vi "Process CAN Frame.vi"(10 "CAN frame":T1 {"type" items=["CAN Data", "CAN Remote"]; "identifier" format="%.0x"}) -> ()   [LabVIEW 2015]
uses:
  <vilib>/RioEmbeddedCAN/RioEmbeddedCAN.llb/CANFrameControl.ctl
  Dashboard/DashDriverInputs.ctl
  MC/MC Temp 1.ctl
  MC/MC Temp 2.ctl
  MC/MC Temp 3.ctl
  MC/MC Position.ctl
  MC/MC Current.ctl
  MC/MC Voltage.ctl
  MC/MC Flux.ctl
  MC/MC Internal Voltages.ctl
  MC/MC State.ctl
  Inverter States.ctl
  Inverter Run Modes.ctl
  VSM States.ctl
  MC/MC Faults.ctl
  MC/MC Torque.ctl
  MC/MC Mod Index and Flux Weakening.ctl
  Global Data.vi
panel:
  in  "Log Unique IDs":bool
  in  "Reset Array":bool
  out "Array":u32[](array[numeric])
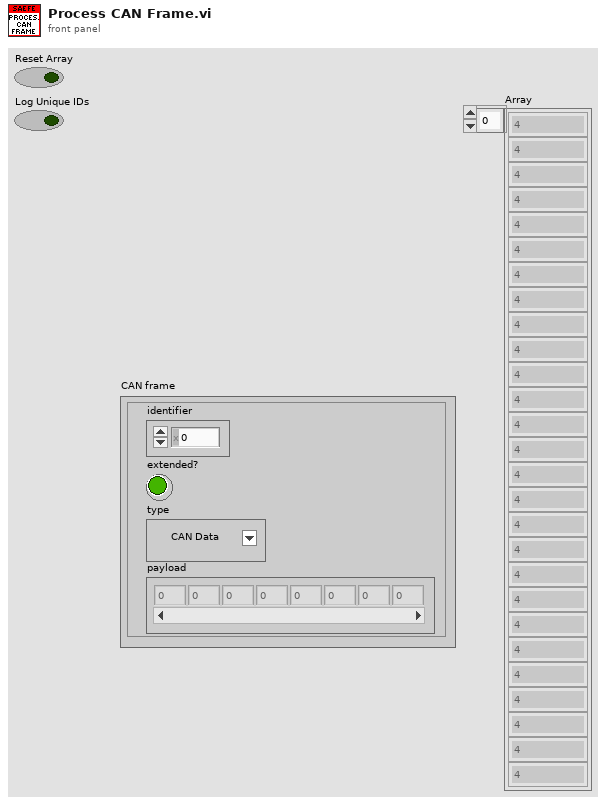
[diagram p1: front panel]
types:
  T1 = typedef "CANFrameControl.ctl" = cluster{"identifier":u32, "extended?":bool, "type":u8, "payload":u8[]}
  T2 = typedef "DashDriverInputs.ctl" = cluster{"ButtonsBitArray":u8, "NRedRotary":u8, "NYellowRotary":u8, "NBlackRotary":u8}
  T3 = typedef "MC Temp 1.ctl" = cluster{"TMCModuleA":dbl, "TMCModuleB":dbl, "TMCModuleC":dbl, "TMCGateDriver":dbl}
  T4 = typedef "MC Temp 2.ctl" = cluster{"TMCControlBoard":dbl, "TMCRTD1":dbl, "TMCRTD2":dbl, "TMCRTD3":dbl}
  T5 = typedef "MC Temp 3.ctl" = cluster{"TMCRTD4":dbl, "TMCRTD5":dbl, "TMotor":dbl, "MTorqueShudder":dbl}
  T6 = typedef "MC Position.ctl" = cluster{"aMotor":dbl, "nMotor":dbl, "fMCOutput":dbl, "aDeltaResolverFilt":dbl}
  T7 = typedef "MC Current.ctl" = cluster{"IMCPhaseA":dbl, "IMCPhaseB":dbl, "IMCPhaseC":dbl, "IMCBatteryCalc":dbl}
  T8 = typedef "MC Voltage.ctl" = cluster{"VMCPhaseAB":dbl, "VMCPhaseBC":dbl, "VMCOutput":dbl, "VMCBattery":dbl}
  T9 = typedef "MC Flux.ctl" = cluster{"IMCFluxCommand":dbl, "IMCFluxFeedback":dbl, "IMC_Id":dbl, "IMC_Iq":dbl}
  T10 = typedef "MC Internal Voltages.ctl" = cluster{"VMCRef1_5":dbl, "VMCRef2_5":dbl, "VMCRef5":dbl, "VMCRef12":dbl}
  T11 = typedef "MC State.ctl" = cluster{"eMCInverterState":T12, "eMCInverterRunMode":T13, "eMCInverterCommandMode":enum16{"CAN Mode", "VSM Mode"}, "bMCInverterEnable":bool, "bMCInverterEnableLockout":bool, "bMCDirectionForward":bool, "eMCVSMState":T14, "bMCRelay1":bool, "bMCRelay2":bool, "bMCRelay3":bool, "bMCRelay4":bool}
  T12 = typedef "Inverter States.ctl" = enum16{"Power On", "Stop", "Open Loop", "Closed Loop", "Wait", "Internal", "Idle Run", "Idle Stop", ""}
  T13 = typedef "Inverter Run Modes.ctl" = enum16{"Torque Mode", "Speed Mode"}
  T14 = typedef "VSM States.ctl" = enum16{"VSM Start", "Pre-Charge Init", "Pre-Charge Active", "Pre-Charge Complete", "VSM Wait", "VSM Ready", "Motor Running", "Blink Fault Code", "Shutdown in Process", "Recycle Power"}
  T15 = typedef "MC Faults.ctl" = cluster{"MC Fault":cluster{"Over-Speed":bool, "Over-Current":bool, "Over-Voltage":bool, "Inverter Over-Temp":bool, "Direction Command":bool, "Inverter Response Time-Out":bool, "Desat Fault":bool, "Hardware Over-Current":bool, "Under-Voltage":bool, "CAN Command Message Lost":bool, "Motor Over-Temp":bool, "Module A Over-Temp":bool, "Module B Over-Temp":bool, "Module C Over-Temp":bool, "PCB Over-Temp":bool, "Gate Driver 1 Over-Temp":bool, "Gate Driver 2 Over-Temp":bool, "Gate Drive 3 Over-Temp":bool, "Current Sensor Fault":bool, "Resolver Not Connected":bool}, "MC Post":u32, "MC RUN":u32}
  T16 = typedef "MC Torque.ctl" = cluster{"MMCRequested":dbl, "MMCFeedback":dbl, "tMCElapsed":u32}
  T17 = typedef "MC Mod Index and Flux Weakening.ctl" = cluster{"NMCModulationIndex":dbl, "IMCFluxWeakeningOutput":dbl, "IMCIdCommand":dbl, "IMCIqCommand":dbl}
  T18 = cluster{"Over-Speed":bool, "Over-Current":bool, "Over-Voltage":bool, "Inverter Over-Temp":bool, "Direction Command":bool, "Inverter Response Time-Out":bool, "Desat Fault":bool, "Hardware Over-Current":bool, "Under-Voltage":bool, "CAN Command Message Lost":bool, "Motor Over-Temp":bool, "Module A Over-Temp":bool, "Module B Over-Temp":bool, "Module C Over-Temp":bool, "PCB Over-Temp":bool, "Gate Driver 1 Over-Temp":bool, "Gate Driver 2 Over-Temp":bool, "Gate Drive 3 Over-Temp":bool, "Current Sensor Fault":bool, "Resolver Not Connected":bool}
  T19 = typedef "BMS Telemetry.ctl" = cluster{"bBMSIgnition":bool, "bBMSChargerMains":bool, "bBMSFastCharge":bool, "bBMSChargerEnabled":bool, "eBMSCarState":enum16{"Off", "On, Not Charging", "Charging", "Charging Finished", "Charging Error"}, "eBMSChargingState":enum16{"Disconnected", "Pre-charging", "Main Charging", "Balancing", "Charging Finished OK", "Charging Error"}, "tBMSChargeStage":u16, "eBMSLastChargeError":enum16{"No Error", "No Cell Communication", "No Cell Communication - Non CAN Charger", "Maximum charging stage duration expired", "Cell Communication Lost during Charge", "Cannot set balancing voltage", "Cell temps too high", "No Comms so can't determine temp", "# of Cells Mismatch", "Cells Overvoltage", "Cell Protection Event occured."}, "NBMSNumCells":u8, "bBMSUnderVProtection":bool, "bBMSOverVProtection":bool, "bBMSOverTProtection":bool, "bBMSLeakageProtection":bool, "bBMSNoCellCommsError":bool, "bBMSLowVReduction":bool, "bBMSHighTReduction":bool, "VCellMin":dbl, "VCellMax":dbl, "VCellMean":dbl, "VTotal":dbl, "TCellMin":dbl, "TCellMax":dbl, "TCellMean":dbl, "VCells":cluster{"[51]":dbl, "[53]":dbl, "[54]":dbl, "[55]":dbl, "[56]":dbl, "[57]":dbl, "[58]":dbl, "[59]":dbl, "[60]":dbl, "[61]":dbl, "[62]":dbl, "[63]":dbl, "[64]":dbl, "[65]":dbl, "[66]":dbl, "[67]":dbl, "[34]":dbl, "[35]":dbl, "[36]":dbl, "[37]":dbl, "[38]":dbl, "[39]":dbl, "[40]":dbl, "[41]":dbl, "[42]":dbl, "[43]":dbl, "[44]":dbl, "[45]":dbl, "[46]":dbl, "[47]":dbl, "[48]":dbl, "[49]":dbl, "[50]":dbl, "[17]":dbl, "[18]":dbl, "[19]":dbl, "[20]":dbl, "[21]":dbl, "[22]":dbl, "[23]":dbl, "[24]":dbl, "[25]":dbl, "[26]":dbl, "[27]":dbl, "[28]":dbl, "[29]":dbl, "[30]":dbl, "[31]":dbl, "[32]":dbl, "[33]":dbl, "[0]":dbl, "[1]":dbl, "[2]":dbl, "[3]":dbl, "[4]":dbl, "[5]":dbl, "[6]":dbl, "[7]":dbl, "[8]":dbl, "[9]":dbl, "[10]":dbl, "[11]":dbl, "[12]":dbl, "[13]":dbl, "[14]":dbl, "[15]":dbl, "[16]":dbl, "[52] 2":dbl}, "TBMSCells":cluster{"[55]":dbl, "[56]":dbl, "[57]":dbl, "[58]":dbl, "[59]":dbl, "[60]":dbl, "[61]":dbl, "[62]":dbl, "[63]":dbl, "[64]":dbl, "[65]":dbl, "[66]":dbl, "[67]":dbl, "[68]":dbl, "[69]":dbl, "[70]":dbl, "[17]":dbl, "[38]":dbl, "[39]":dbl, "[40]":dbl, "[41]":dbl, "[42]":dbl, "[43]":dbl, "[44]":dbl, "[45]":dbl, "[46]":dbl, "[47]":dbl, "[48]":dbl, "[49]":dbl, "[50]":dbl, "[51]":dbl, "[52]":dbl, "[53]":dbl, "[54]":dbl, "[21]":dbl, "[22]":dbl, "[23]":dbl, "[24]":dbl, "[25]":dbl, "[26]":dbl, "[27]":dbl, "[28]":dbl, "[29]":dbl, "[30]":dbl, "[31]":dbl, "[32]":dbl, "[33]":dbl, "[34]":dbl, "[35]":dbl, "[36]":dbl, "[37]":dbl, "[0]":dbl, "[1]":dbl, "[2]":dbl, "[3]":dbl, "[4]":dbl, "[5]":dbl, "[6]":dbl, "[7]":dbl, "[8]":dbl, "[9]":dbl, "[10]":dbl, "[11]":dbl, "[12]":dbl, "[13]":dbl, "[14]":dbl, "[15]":dbl, "[16]":dbl}, "bChargerConnected":bool, "VChargerSetpoint":dbl, "IChargerSetpoint":dbl, "VChargerActual":dbl, "IChargerActual":dbl, "BCells":cluster{"[51]":dbl, "[52]":dbl, "[53]":dbl, "[54]":dbl, "[55]":dbl, "[56]":dbl, "[57]":dbl, "[58]":dbl, "[59]":dbl, "[60]":dbl, "[61]":dbl, "[62]":dbl, "[63]":dbl, "[64]":dbl, "[65]":dbl, "[66]":dbl, "[67]":dbl, "[34]":dbl, "[35]":dbl, "[36]":dbl, "[37]":dbl, "[38]":dbl, "[39]":dbl, "[40]":dbl, "[41]":dbl, "[42]":dbl, "[43]":dbl, "[44]":dbl, "[45]":dbl, "[46]":dbl, "[47]":dbl, "[48]":dbl, "[49]":dbl, "[50]":dbl, "[17]":dbl, "[18]":dbl, "[19]":dbl, "[20]":dbl, "[21]":dbl, "[22]":dbl, "[23]":dbl, "[24]":dbl, "[25]":dbl, "[26]":dbl, "[27]":dbl, "[28]":dbl, "[29]":dbl, "[30]":dbl, "[31]":dbl, "[32]":dbl, "[33]":dbl, "[0]":dbl, "[1]":dbl, "[2]":dbl, "[3]":dbl, "[4]":dbl, "[5]":dbl, "[6]":dbl, "[7]":dbl, "[8]":dbl, "[9]":dbl, "[10]":dbl, "[11]":dbl, "[12]":dbl, "[13]":dbl, "[14]":dbl, "[15]":dbl, "[16]":dbl}, "bNewVCellMinSample":bool, "Battery Temp":cluster{"[0]":dbl, "[1]":dbl, "[2]":dbl, "[3]":dbl, "[4]":dbl, "[5]":dbl, "[6]":dbl, "[7]":dbl, "[8]":dbl, "[9]":dbl, "[10]":dbl, "[11]":dbl, "[12]":dbl, "[13]":dbl, "[14]":dbl, "[15]":dbl, "[16]":dbl, "[17]":dbl, "[18]":dbl, "[19]":dbl, "[20]":dbl, "[21]":dbl, "[22]":dbl, "[23]":dbl, "[24]":dbl, "[25]":dbl, "[26]":dbl, "[27]":dbl, "[28]":dbl, "[29]":dbl, "[30]":dbl, "[31]":dbl, "[32]":dbl, "[33]":dbl, "[34]":dbl, "[35]":dbl, "[36]":dbl, "[37]":dbl, "[38]":dbl, "[39]":dbl, "[40]":dbl, "[41]":dbl, "[42]":dbl, "[43]":dbl, "[44]":dbl, "[45]":dbl, "[46]":dbl, "[47]":dbl, "[48]":dbl, "[49]":dbl, "[50]":dbl, "[51]":dbl, "[52]":dbl, "[53]":dbl, "[54]":dbl, "[55]":dbl, "[56]":dbl, "[57]":dbl, "[58]":dbl, "[59]":dbl, "[60]":dbl, "[61]":dbl, "[62]":dbl, "[63]":dbl, "[64]":dbl, "[65]":dbl, "[66]":dbl, "[67]":dbl, "[68]":dbl, "[69]":dbl, "[71]":dbl, "[70]":dbl, "[0] 2":dbl, "[1] 2":dbl, "[2] 2":dbl, "[3] 2":dbl, "[4] 2":dbl, "[5] 2":dbl, "[6] 2":dbl, "[7] 2":dbl, "[8] 2":dbl, "[9] 2":dbl, "[10] 2":dbl, "[11] 2":dbl, "[12] 2":dbl, "[13] 2":dbl, "[14] 2":dbl, "[15] 2":dbl, "[16] 2":dbl, "[17] 2":dbl, "[18] 2":dbl, "[19] 2":dbl, "[20] 2":dbl, "[21] 2":dbl, "[22] 2":dbl, "[23] 2":dbl, "[24] 2":dbl, "[25] 2":dbl, "[26] 2":dbl, "[27] 2":dbl, "[28] 2":dbl, "[29] 2":dbl, "[30] 2":dbl, "[31] 2":dbl, "[32] 2":dbl, "[33] 2":dbl, "[34] 2":dbl, "[35] 2":dbl, "[36] 2":dbl, "[37] 2":dbl, "[38] 2":dbl, "[39] 2":dbl, "[40] 2":dbl, "[41] 2":dbl, "[42] 2":dbl, "[43] 2":dbl, "[44] 2":dbl, "[45] 2":dbl, "[46] 2":dbl, "[47] 2":dbl, "[48] 2":dbl, "[49] 2":dbl, "[50] 2":dbl, "[51] 2":dbl, "[52] 3":dbl, "[53] 2":dbl, "[54] 2":dbl, "[55] 2":dbl, "[56] 2":dbl, "[57] 2":dbl, "[58] 2":dbl, "[59] 2":dbl, "[60] 2":dbl, "[61] 2":dbl, "[62] 2":dbl, "[63] 2":dbl, "[64] 2":dbl, "[65] 2":dbl, "[66] 2":dbl, "[67] 2":dbl, "[68]2":dbl, "[69]2":dbl, "[70]2":dbl, "[71]2":dbl, "[0] 3":dbl, "[1] 3":dbl, "[2] 3":dbl, "[3] 3":dbl, "[4] 3":dbl, "[5] 3":dbl, "[6] 3":dbl, "[7] 3":dbl, "[8] 3":dbl, "[9] 3":dbl, "[10] 3":dbl, "[11] 3":dbl, "[12] 3":dbl, "[13] 3":dbl, "[14] 3":dbl, "[15] 3":dbl, "[16] 3":dbl, "[17] 3":dbl, "[18] 3":dbl, "[19] 3":dbl, "[20] 3":dbl, "[21] 3":dbl, "[22] 3":dbl, "[23] 3":dbl, "[24] 3":dbl, "[25] 3":dbl, "[26] 3":dbl, "[27] 3":dbl, "[28] 3":dbl, "[29] 3":dbl, "[30] 3":dbl, "[31] 3":dbl, "[32] 3":dbl, "[33] 3":dbl, "[34] 3":dbl, "[35] 3":dbl, "[36] 3":dbl, "[37] 3":dbl, "[38] 3":dbl, "[39] 3":dbl, "[40] 3":dbl, "[41] 3":dbl, "[42] 3":dbl, "[43] 3":dbl, "[44] 3":dbl, "[45] 3":dbl, "[46] 3":dbl, "[47] 3":dbl, "[48] 3":dbl, "[49] 3":dbl, "[50] 3":dbl, "[51] 3":dbl, "[52] 4":dbl, "[53] 3":dbl, "[54] 3":dbl, "[55] 3":dbl, "[56] 3":dbl, "[57] 3":dbl, "[58] 3":dbl, "[59] 3":dbl, "[60] 3":dbl, "[61] 3":dbl, "[62] 3":dbl, "[63] 3":dbl, "[64] 3":dbl, "[65] 3":dbl, "[66] 3":dbl, "[67] 3":dbl, "[68]3":dbl, "[69]3":dbl, "[70]3":dbl, "[71]3":dbl, "[4] 4":dbl, "[5] 4":dbl, "[6] 4":dbl, "[7] 4":dbl, "[8] 4":dbl, "[9] 4":dbl, "[10] 4":dbl, "[11] 4":dbl, "[12] 4":dbl, "[13] 4":dbl, "[14] 4":dbl, "[15] 4":dbl, "[16] 4":dbl, "[17] 4":dbl, "[18] 4":dbl, "[19] 4":dbl, "[20] 4":dbl, "[21] 4":dbl, "[22] 4":dbl, "[23] 4":dbl, "[24] 4":dbl, "[25] 4":dbl, "[26] 4":dbl, "[27] 4":dbl, "[28] 4":dbl, "[29] 4":dbl, "[30] 4":dbl, "[31] 4":dbl, "[32] 4":dbl, "[33] 4":dbl, "[17] 9":dbl, "[0] 9":dbl, "[51] 8":dbl, "[34] 8":dbl, "[17] 8":dbl, "[0] 8":dbl, "[34] 4":dbl, "[35] 4":dbl, "[36] 4":dbl, "[37] 4":dbl, "[38] 4":dbl, "[39] 4":dbl, "[40] 4":dbl, "[41] 4":dbl, "[42] 4":dbl, "[43] 4":dbl, "[44] 4":dbl, "[45] 4":dbl, "[46] 4":dbl, "[47] 4":dbl, "[48] 4":dbl, "[49] 4":dbl, "[50] 4":dbl, "[34] 9":dbl, "[51] 4":dbl, "[52] 5":dbl, "[53] 4":dbl, "[54] 4":dbl, "[55] 4":dbl, "[56] 4":dbl, "[57] 4":dbl, "[58] 4":dbl, "[59] 4":dbl, "[60] 4":dbl, "[61] 4":dbl, "[62] 4":dbl, "[63] 4":dbl, "[64] 4":dbl, "[65] 4":dbl, "[66] 4":dbl, "[67] 4":dbl, "[51] 9":dbl}, "TBMSMax":dbl, "TBMSMin":dbl, "TBMSMean":dbl}
  T20 = enum16{"Off", "On, Not Charging", "Charging", "Charging Finished", "Charging Error"}
  T21 = enum16{"Disconnected", "Pre-charging", "Main Charging", "Balancing", "Charging Finished OK", "Charging Error"}
  T22 = cluster{"[51]":dbl, "[53]":dbl, "[54]":dbl, "[55]":dbl, "[56]":dbl, "[57]":dbl, "[58]":dbl, "[59]":dbl, "[60]":dbl, "[61]":dbl, "[62]":dbl, "[63]":dbl, "[64]":dbl, "[65]":dbl, "[66]":dbl, "[67]":dbl, "[34]":dbl, "[35]":dbl, "[36]":dbl, "[37]":dbl, "[38]":dbl, "[39]":dbl, "[40]":dbl, "[41]":dbl, "[42]":dbl, "[43]":dbl, "[44]":dbl, "[45]":dbl, "[46]":dbl, "[47]":dbl, "[48]":dbl, "[49]":dbl, "[50]":dbl, "[17]":dbl, "[18]":dbl, "[19]":dbl, "[20]":dbl, "[21]":dbl, "[22]":dbl, "[23]":dbl, "[24]":dbl, "[25]":dbl, "[26]":dbl, "[27]":dbl, "[28]":dbl, "[29]":dbl, "[30]":dbl, "[31]":dbl, "[32]":dbl, "[33]":dbl, "[0]":dbl, "[1]":dbl, "[2]":dbl, "[3]":dbl, "[4]":dbl, "[5]":dbl, "[6]":dbl, "[7]":dbl, "[8]":dbl, "[9]":dbl, "[10]":dbl, "[11]":dbl, "[12]":dbl, "[13]":dbl, "[14]":dbl, "[15]":dbl, "[16]":dbl, "[52] 2":dbl}
  T23 = cluster{"VCells[0]":dbl, "VCells[1]":dbl, "VCells[2]":dbl, "VCells[3]":dbl, "VCells[4]":dbl, "VCells[5]":dbl, "VCells[6]":dbl, "VCells[7]":dbl, "VCells[8]":dbl, "VCells[9]":dbl, "VCells[10]":dbl, "VCells[11]":dbl, "VCells[12]":dbl, "VCells[13]":dbl, "VCells[14]":dbl, "VCells[15]":dbl, "VCells[16]":dbl, "VCells[17]":dbl, "VCells[18]":dbl, "VCells[19]":dbl, "VCells[20]":dbl, "VCells[21]":dbl, "VCells[22]":dbl, "VCells[23]":dbl, "VCells[24]":dbl, "VCells[25]":dbl, "VCells[26]":dbl, "VCells[27]":dbl, "VCells[28]":dbl, "VCells[29]":dbl, "VCells[30]":dbl, "VCells[31]":dbl, "VCells[32]":dbl, "VCells[33]":dbl, "VCells[34]":dbl, "VCells[35]":dbl, "VCells[36]":dbl, "VCells[37]":dbl, "VCells[38]":dbl, "VCells[39]":dbl, "VCells[40]":dbl, "VCells[41]":dbl, "VCells[42]":dbl, "VCells[43]":dbl, "VCells[44]":dbl, "VCells[45]":dbl, "VCells[46]":dbl, "VCells[47]":dbl, "VCells[48]":dbl, "VCells[49]":dbl, "VCells[50]":dbl, "VCells[51]":dbl, "VCells[52]":dbl, "VCells[53]":dbl, "VCells[54]":dbl, "VCells[55]":dbl, "VCells[56]":dbl, "VCells[57]":dbl, "VCells[58]":dbl, "VCells[59]":dbl, "VCells[60]":dbl, "VCells[61]":dbl, "VCells[62]":dbl, "VCells[63]":dbl, "VCells[64]":dbl, "VCells[65]":dbl, "VCells[66]":dbl, "VCells[67]":dbl}
  T24 = cluster{"[55]":dbl, "[56]":dbl, "[57]":dbl, "[58]":dbl, "[59]":dbl, "[60]":dbl, "[61]":dbl, "[62]":dbl, "[63]":dbl, "[64]":dbl, "[65]":dbl, "[66]":dbl, "[67]":dbl, "[68]":dbl, "[69]":dbl, "[70]":dbl, "[17]":dbl, "[38]":dbl, "[39]":dbl, "[40]":dbl, "[41]":dbl, "[42]":dbl, "[43]":dbl, "[44]":dbl, "[45]":dbl, "[46]":dbl, "[47]":dbl, "[48]":dbl, "[49]":dbl, "[50]":dbl, "[51]":dbl, "[52]":dbl, "[53]":dbl, "[54]":dbl, "[21]":dbl, "[22]":dbl, "[23]":dbl, "[24]":dbl, "[25]":dbl, "[26]":dbl, "[27]":dbl, "[28]":dbl, "[29]":dbl, "[30]":dbl, "[31]":dbl, "[32]":dbl, "[33]":dbl, "[34]":dbl, "[35]":dbl, "[36]":dbl, "[37]":dbl, "[0]":dbl, "[1]":dbl, "[2]":dbl, "[3]":dbl, "[4]":dbl, "[5]":dbl, "[6]":dbl, "[7]":dbl, "[8]":dbl, "[9]":dbl, "[10]":dbl, "[11]":dbl, "[12]":dbl, "[13]":dbl, "[14]":dbl, "[15]":dbl, "[16]":dbl}
  T25 = cluster{"TBMSCells[0]":dbl, "TBMSCells[1]":dbl, "TBMSCells[2]":dbl, "TBMSCells[3]":dbl, "TBMSCells[4]":dbl, "TBMSCells[5]":dbl, "TBMSCells[6]":dbl, "TBMSCells[7]":dbl, "TBMSCells[8]":dbl, "TBMSCells[9]":dbl, "TBMSCells[10]":dbl, "TBMSCells[11]":dbl, "TBMSCells[12]":dbl, "TBMSCells[13]":dbl, "TBMSCells[14]":dbl, "TBMSCells[15]":dbl, "TBMSCells[16]":dbl, "TBMSCells[17]":dbl, "TBMSCells[18]":dbl, "TBMSCells[19]":dbl, "TBMSCells[20]":dbl, "TBMSCells[21]":dbl, "TBMSCells[22]":dbl, "TBMSCells[23]":dbl, "TBMSCells[24]":dbl, "TBMSCells[25]":dbl, "TBMSCells[26]":dbl, "TBMSCells[27]":dbl, "TBMSCells[28]":dbl, "TBMSCells[29]":dbl, "TBMSCells[30]":dbl, "TBMSCells[31]":dbl, "TBMSCells[32]":dbl, "TBMSCells[33]":dbl, "TBMSCells[34]":dbl, "TBMSCells[35]":dbl, "TBMSCells[36]":dbl, "TBMSCells[37]":dbl, "TBMSCells[38]":dbl, "TBMSCells[39]":dbl, "TBMSCells[40]":dbl, "TBMSCells[41]":dbl, "TBMSCells[42]":dbl, "TBMSCells[43]":dbl, "TBMSCells[44]":dbl, "TBMSCells[45]":dbl, "TBMSCells[46]":dbl, "TBMSCells[47]":dbl, "TBMSCells[48]":dbl, "TBMSCells[49]":dbl, "TBMSCells[50]":dbl, "TBMSCells[51]":dbl, "TBMSCells[52]":dbl, "TBMSCells[53]":dbl, "TBMSCells[54]":dbl, "TBMSCells[55]":dbl, "TBMSCells[56]":dbl, "TBMSCells[57]":dbl, "TBMSCells[58]":dbl, "TBMSCells[59]":dbl, "TBMSCells[60]":dbl, "TBMSCells[61]":dbl, "TBMSCells[62]":dbl, "TBMSCells[63]":dbl, "TBMSCells[64]":dbl, "TBMSCells[65]":dbl, "TBMSCells[66]":dbl, "TBMSCells[67]":dbl}
  T26 = cluster{"[51]":dbl, "[52]":dbl, "[53]":dbl, "[54]":dbl, "[55]":dbl, "[56]":dbl, "[57]":dbl, "[58]":dbl, "[59]":dbl, "[60]":dbl, "[61]":dbl, "[62]":dbl, "[63]":dbl, "[64]":dbl, "[65]":dbl, "[66]":dbl, "[67]":dbl, "[34]":dbl, "[35]":dbl, "[36]":dbl, "[37]":dbl, "[38]":dbl, "[39]":dbl, "[40]":dbl, "[41]":dbl, "[42]":dbl, "[43]":dbl, "[44]":dbl, "[45]":dbl, "[46]":dbl, "[47]":dbl, "[48]":dbl, "[49]":dbl, "[50]":dbl, "[17]":dbl, "[18]":dbl, "[19]":dbl, "[20]":dbl, "[21]":dbl, "[22]":dbl, "[23]":dbl, "[24]":dbl, "[25]":dbl, "[26]":dbl, "[27]":dbl, "[28]":dbl, "[29]":dbl, "[30]":dbl, "[31]":dbl, "[32]":dbl, "[33]":dbl, "[0]":dbl, "[1]":dbl, "[2]":dbl, "[3]":dbl, "[4]":dbl, "[5]":dbl, "[6]":dbl, "[7]":dbl, "[8]":dbl, "[9]":dbl, "[10]":dbl, "[11]":dbl, "[12]":dbl, "[13]":dbl, "[14]":dbl, "[15]":dbl, "[16]":dbl}
  T27 = cluster{"BCells[0]":dbl, "BCells[1]":dbl, "BCells[2]":dbl, "BCells[3]":dbl, "BCells[4]":dbl, "BCells[5]":dbl, "BCells[6]":dbl, "BCells[7]":dbl, "BCells[8]":dbl, "BCells[9]":dbl, "BCells[10]":dbl, "BCells[11]":dbl, "BCells[12]":dbl, "BCells[13]":dbl, "BCells[14]":dbl, "BCells[15]":dbl, "BCells[16]":dbl, "BCells[17]":dbl, "BCells[18]":dbl, "BCells[19]":dbl, "BCells[20]":dbl, "BCells[21]":dbl, "BCells[22]":dbl, "BCells[23]":dbl, "BCells[24]":dbl, "BCells[25]":dbl, "BCells[26]":dbl, "BCells[27]":dbl, "BCells[28]":dbl, "BCells[29]":dbl, "BCells[30]":dbl, "BCells[31]":dbl, "BCells[32]":dbl, "BCells[33]":dbl, "BCells[34]":dbl, "BCells[35]":dbl, "BCells[36]":dbl, "BCells[37]":dbl, "BCells[38]":dbl, "BCells[39]":dbl, "BCells[40]":dbl, "BCells[41]":dbl, "BCells[42]":dbl, "BCells[43]":dbl, "BCells[44]":dbl, "BCells[45]":dbl, "BCells[46]":dbl, "BCells[47]":dbl, "BCells[48]":dbl, "BCells[49]":dbl, "BCells[50]":dbl, "BCells[51]":dbl, "BCells[52]":dbl, "BCells[53]":dbl, "BCells[54]":dbl, "BCells[55]":dbl, "BCells[56]":dbl, "BCells[57]":dbl, "BCells[58]":dbl, "BCells[59]":dbl, "BCells[60]":dbl, "BCells[61]":dbl, "BCells[62]":dbl, "BCells[63]":dbl, "BCells[64]":dbl, "BCells[65]":dbl, "BCells[66]":dbl, "BCells[67]":dbl}
  T28 = cluster{dbl, dbl, dbl, dbl, dbl, dbl, dbl, dbl, dbl, dbl, dbl, dbl, dbl, dbl, dbl, dbl, dbl, dbl, dbl, dbl, dbl, dbl, dbl, dbl, dbl, dbl, dbl, dbl, dbl, dbl, dbl, dbl, dbl, dbl, dbl, dbl, dbl, dbl, dbl, dbl, dbl, dbl, dbl, dbl, dbl, dbl, dbl, dbl, dbl, dbl, dbl, dbl, dbl, dbl, dbl, dbl, dbl, dbl, dbl, dbl, dbl, dbl, dbl, dbl, dbl, dbl, dbl, dbl, dbl, dbl, dbl, dbl, dbl, dbl, dbl, dbl, dbl, dbl, dbl, dbl, dbl, dbl, dbl, dbl, dbl, dbl, dbl, dbl, dbl, dbl, dbl, dbl, dbl, dbl, dbl, dbl, dbl, dbl, dbl, dbl, dbl, dbl, dbl, dbl, dbl, dbl, dbl, dbl, dbl, dbl, dbl, dbl, dbl, dbl, dbl, dbl, dbl, dbl, dbl, dbl, dbl, dbl, dbl, dbl, dbl, dbl, dbl, dbl, dbl, dbl, dbl, dbl, dbl, dbl, dbl, dbl, dbl, dbl, dbl, dbl, dbl, dbl, dbl, dbl, dbl, dbl, dbl, dbl, dbl, dbl, dbl, dbl, dbl, dbl, dbl, dbl, dbl, dbl, dbl, dbl, dbl, dbl, dbl, dbl, dbl, dbl, dbl, dbl, dbl, dbl, dbl, dbl, dbl, dbl, dbl, dbl, dbl, dbl, dbl, dbl, dbl, dbl, dbl, dbl, dbl, dbl, dbl, dbl, dbl, dbl, dbl, dbl, dbl, dbl, dbl, dbl, dbl, dbl, dbl, dbl, dbl, dbl, dbl, dbl, dbl, dbl, dbl, dbl, dbl, dbl, dbl, dbl, dbl, dbl, dbl, dbl, dbl, dbl, dbl, dbl, dbl, dbl, dbl, dbl, dbl, dbl, dbl, dbl, dbl, dbl, dbl, dbl, dbl, dbl, dbl, dbl, dbl, dbl, dbl, dbl, dbl, dbl, dbl, dbl, dbl, dbl, dbl, dbl, dbl, dbl, dbl, dbl, dbl, dbl, dbl, dbl, dbl, dbl, dbl, dbl, dbl, dbl, dbl, dbl, dbl, dbl, dbl, dbl, dbl, dbl, dbl, dbl, dbl, dbl, dbl, dbl, dbl, dbl, dbl, dbl, dbl, dbl, dbl, dbl, dbl, dbl, dbl, dbl}
  T29 = cluster{"[0]":dbl, "[1]":dbl, "[2]":dbl, "[3]":dbl, "[4]":dbl, "[5]":dbl, "[6]":dbl, "[7]":dbl, "[8]":dbl, "[9]":dbl, "[10]":dbl, "[11]":dbl, "[12]":dbl, "[13]":dbl, "[14]":dbl, "[15]":dbl, "[16]":dbl, "[17]":dbl, "[18]":dbl, "[19]":dbl, "[20]":dbl, "[21]":dbl, "[22]":dbl, "[23]":dbl, "[24]":dbl, "[25]":dbl, "[26]":dbl, "[27]":dbl, "[28]":dbl, "[29]":dbl, "[30]":dbl, "[31]":dbl, "[32]":dbl, "[33]":dbl, "[34]":dbl, "[35]":dbl, "[36]":dbl, "[37]":dbl, "[38]":dbl, "[39]":dbl, "[40]":dbl, "[41]":dbl, "[42]":dbl, "[43]":dbl, "[44]":dbl, "[45]":dbl, "[46]":dbl, "[47]":dbl, "[48]":dbl, "[49]":dbl, "[50]":dbl, "[51]":dbl, "[52]":dbl, "[53]":dbl, "[54]":dbl, "[55]":dbl, "[56]":dbl, "[57]":dbl, "[58]":dbl, "[59]":dbl, "[60]":dbl, "[61]":dbl, "[62]":dbl, "[63]":dbl, "[64]":dbl, "[65]":dbl, "[66]":dbl, "[67]":dbl, "[68]":dbl, "[69]":dbl, "[71]":dbl, "[70]":dbl, "[0] 2":dbl, "[1] 2":dbl, "[2] 2":dbl, "[3] 2":dbl, "[4] 2":dbl, "[5] 2":dbl, "[6] 2":dbl, "[7] 2":dbl, "[8] 2":dbl, "[9] 2":dbl, "[10] 2":dbl, "[11] 2":dbl, "[12] 2":dbl, "[13] 2":dbl, "[14] 2":dbl, "[15] 2":dbl, "[16] 2":dbl, "[17] 2":dbl, "[18] 2":dbl, "[19] 2":dbl, "[20] 2":dbl, "[21] 2":dbl, "[22] 2":dbl, "[23] 2":dbl, "[24] 2":dbl, "[25] 2":dbl, "[26] 2":dbl, "[27] 2":dbl, "[28] 2":dbl, "[29] 2":dbl, "[30] 2":dbl, "[31] 2":dbl, "[32] 2":dbl, "[33] 2":dbl, "[34] 2":dbl, "[35] 2":dbl, "[36] 2":dbl, "[37] 2":dbl, "[38] 2":dbl, "[39] 2":dbl, "[40] 2":dbl, "[41] 2":dbl, "[42] 2":dbl, "[43] 2":dbl, "[44] 2":dbl, "[45] 2":dbl, "[46] 2":dbl, "[47] 2":dbl, "[48] 2":dbl, "[49] 2":dbl, "[50] 2":dbl, "[51] 2":dbl, "[52] 3":dbl, "[53] 2":dbl, "[54] 2":dbl, "[55] 2":dbl, "[56] 2":dbl, "[57] 2":dbl, "[58] 2":dbl, "[59] 2":dbl, "[60] 2":dbl, "[61] 2":dbl, "[62] 2":dbl, "[63] 2":dbl, "[64] 2":dbl, "[65] 2":dbl, "[66] 2":dbl, "[67] 2":dbl, "[68]2":dbl, "[69]2":dbl, "[70]2":dbl, "[71]2":dbl, "[0] 3":dbl, "[1] 3":dbl, "[2] 3":dbl, "[3] 3":dbl, "[4] 3":dbl, "[5] 3":dbl, "[6] 3":dbl, "[7] 3":dbl, "[8] 3":dbl, "[9] 3":dbl, "[10] 3":dbl, "[11] 3":dbl, "[12] 3":dbl, "[13] 3":dbl, "[14] 3":dbl, "[15] 3":dbl, "[16] 3":dbl, "[17] 3":dbl, "[18] 3":dbl, "[19] 3":dbl, "[20] 3":dbl, "[21] 3":dbl, "[22] 3":dbl, "[23] 3":dbl, "[24] 3":dbl, "[25] 3":dbl, "[26] 3":dbl, "[27] 3":dbl, "[28] 3":dbl, "[29] 3":dbl, "[30] 3":dbl, "[31] 3":dbl, "[32] 3":dbl, "[33] 3":dbl, "[34] 3":dbl, "[35] 3":dbl, "[36] 3":dbl, "[37] 3":dbl, "[38] 3":dbl, "[39] 3":dbl, "[40] 3":dbl, "[41] 3":dbl, "[42] 3":dbl, "[43] 3":dbl, "[44] 3":dbl, "[45] 3":dbl, "[46] 3":dbl, "[47] 3":dbl, "[48] 3":dbl, "[49] 3":dbl, "[50] 3":dbl, "[51] 3":dbl, "[52] 4":dbl, "[53] 3":dbl, "[54] 3":dbl, "[55] 3":dbl, "[56] 3":dbl, "[57] 3":dbl, "[58] 3":dbl, "[59] 3":dbl, "[60] 3":dbl, "[61] 3":dbl, "[62] 3":dbl, "[63] 3":dbl, "[64] 3":dbl, "[65] 3":dbl, "[66] 3":dbl, "[67] 3":dbl, "[68]3":dbl, "[69]3":dbl, "[70]3":dbl, "[71]3":dbl, "[4] 4":dbl, "[5] 4":dbl, "[6] 4":dbl, "[7] 4":dbl, "[8] 4":dbl, "[9] 4":dbl, "[10] 4":dbl, "[11] 4":dbl, "[12] 4":dbl, "[13] 4":dbl, "[14] 4":dbl, "[15] 4":dbl, "[16] 4":dbl, "[17] 4":dbl, "[18] 4":dbl, "[19] 4":dbl, "[20] 4":dbl, "[21] 4":dbl, "[22] 4":dbl, "[23] 4":dbl, "[24] 4":dbl, "[25] 4":dbl, "[26] 4":dbl, "[27] 4":dbl, "[28] 4":dbl, "[29] 4":dbl, "[30] 4":dbl, "[31] 4":dbl, "[32] 4":dbl, "[33] 4":dbl, "[17] 9":dbl, "[0] 9":dbl, "[51] 8":dbl, "[34] 8":dbl, "[17] 8":dbl, "[0] 8":dbl, "[34] 4":dbl, "[35] 4":dbl, "[36] 4":dbl, "[37] 4":dbl, "[38] 4":dbl, "[39] 4":dbl, "[40] 4":dbl, "[41] 4":dbl, "[42] 4":dbl, "[43] 4":dbl, "[44] 4":dbl, "[45] 4":dbl, "[46] 4":dbl, "[47] 4":dbl, "[48] 4":dbl, "[49] 4":dbl, "[50] 4":dbl, "[34] 9":dbl, "[51] 4":dbl, "[52] 5":dbl, "[53] 4":dbl, "[54] 4":dbl, "[55] 4":dbl, "[56] 4":dbl, "[57] 4":dbl, "[58] 4":dbl, "[59] 4":dbl, "[60] 4":dbl, "[61] 4":dbl, "[62] 4":dbl, "[63] 4":dbl, "[64] 4":dbl, "[65] 4":dbl, "[66] 4":dbl, "[67] 4":dbl, "[51] 9":dbl}
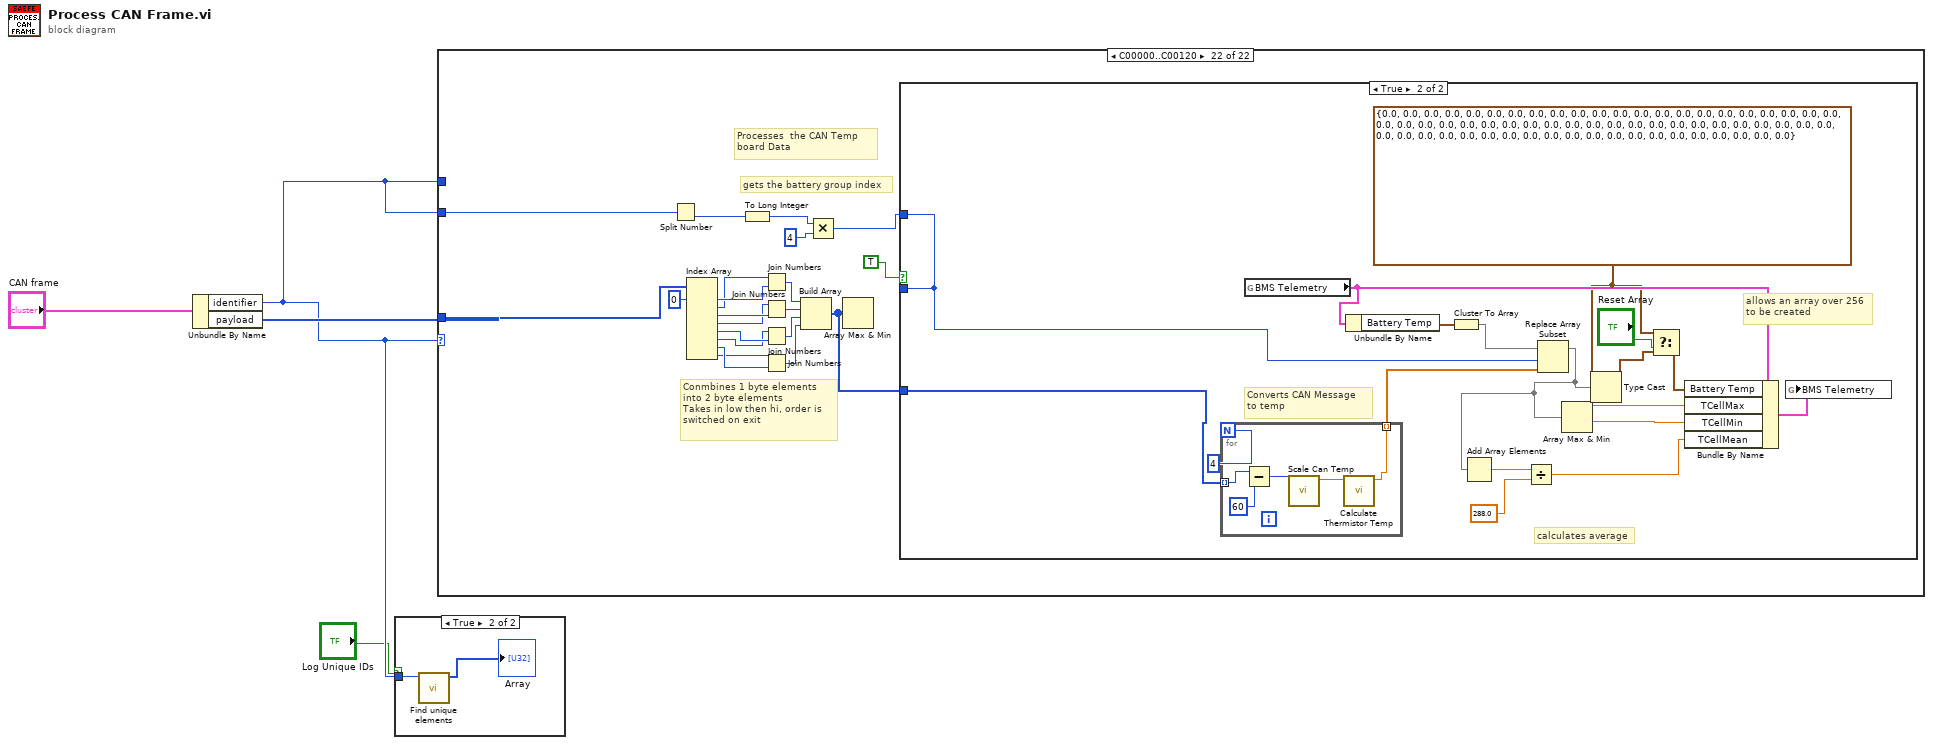
[diagram p0: block diagram]
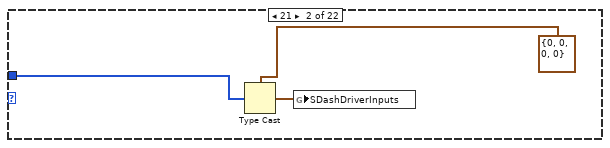
[diagram p4: hidden frame]
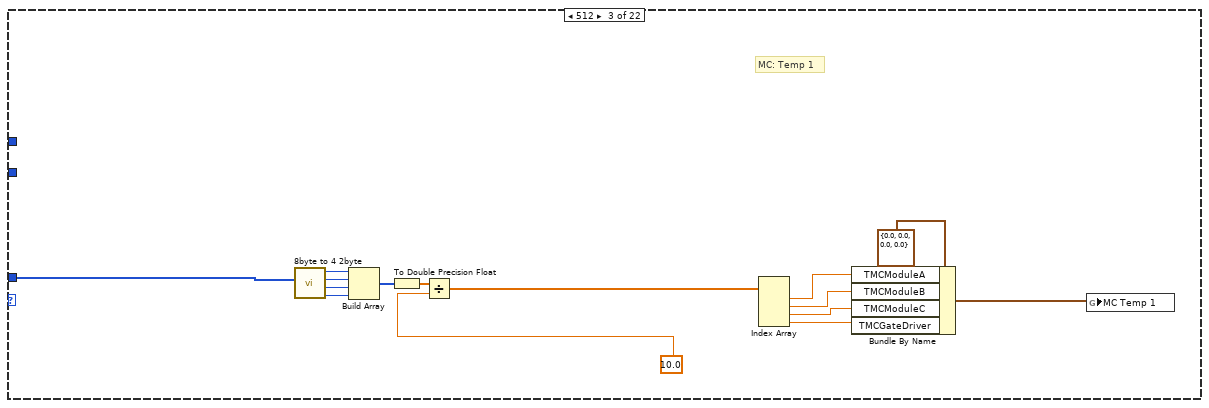
[diagram p5: hidden frame]
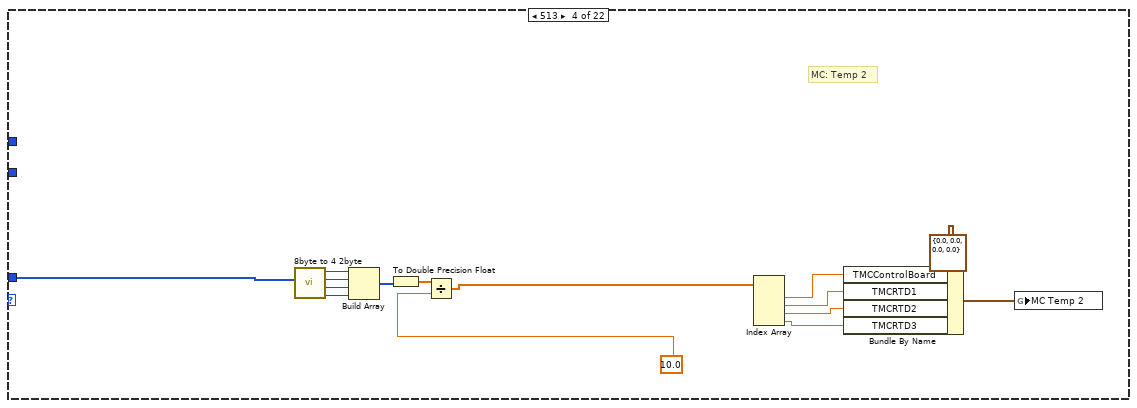
[diagram p6: hidden frame]
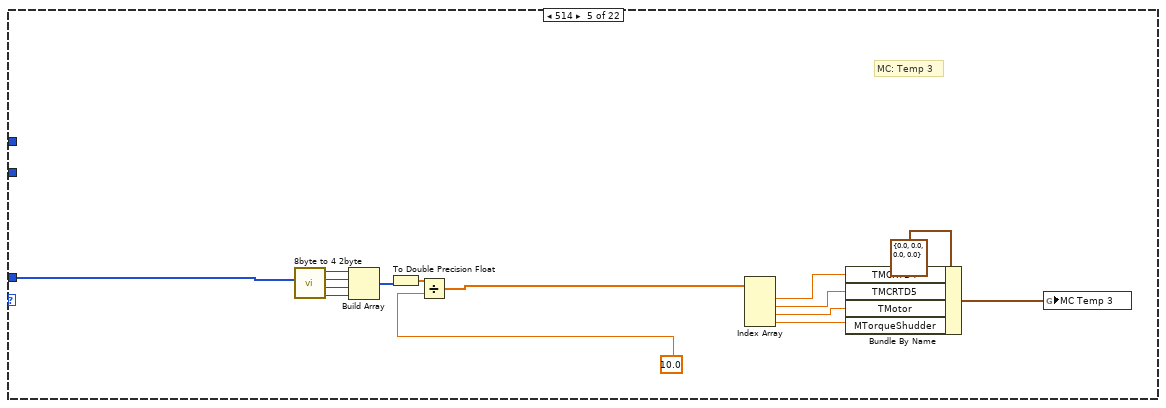
[diagram p7: hidden frame]
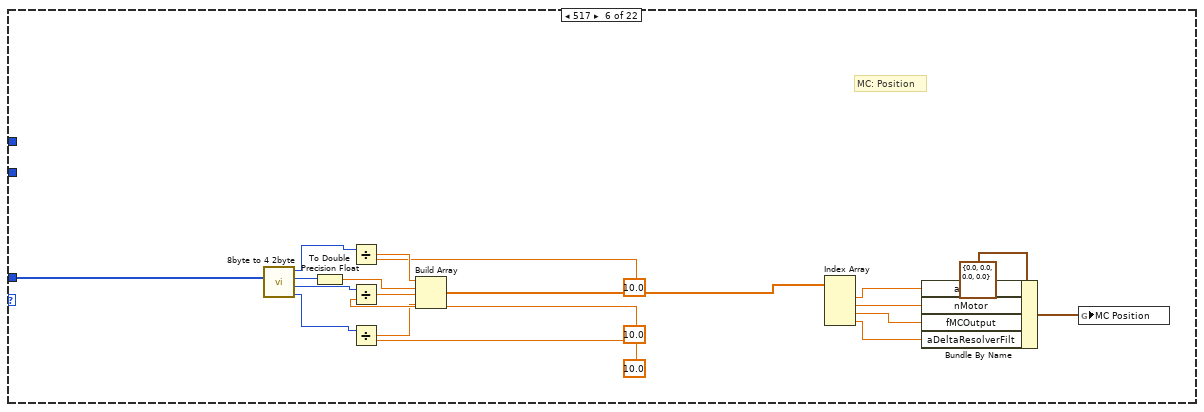
[diagram p8: hidden frame]
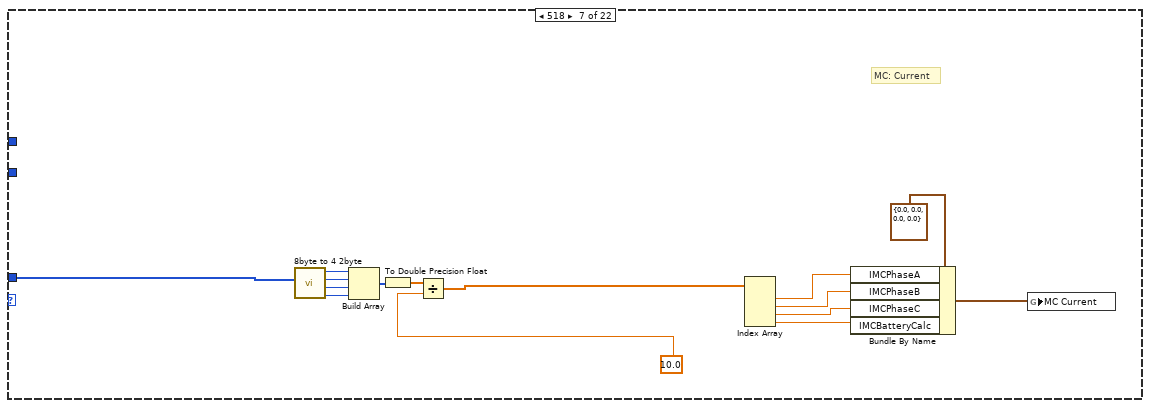
[diagram p9: hidden frame]
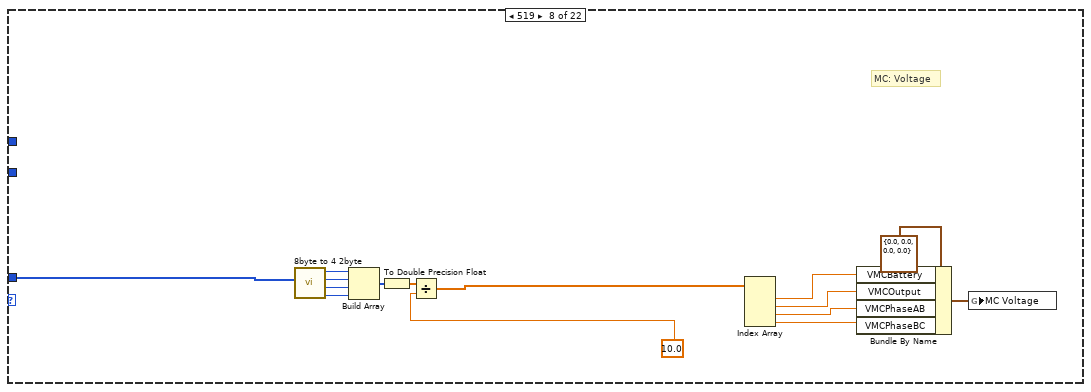
[diagram p10: hidden frame]
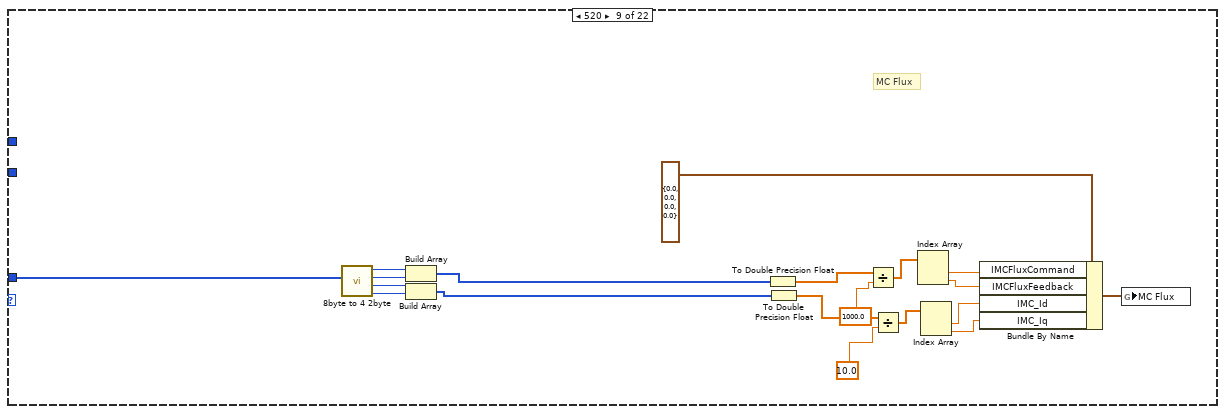
[diagram p11: hidden frame]
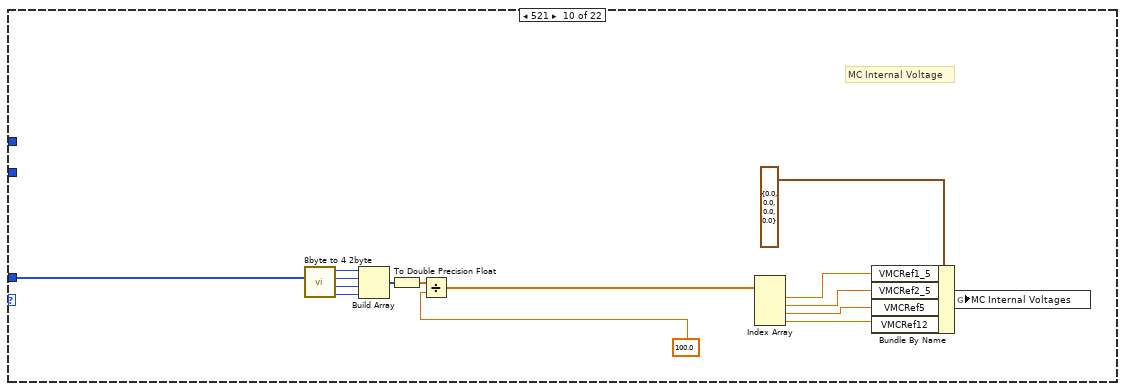
[diagram p12: hidden frame]
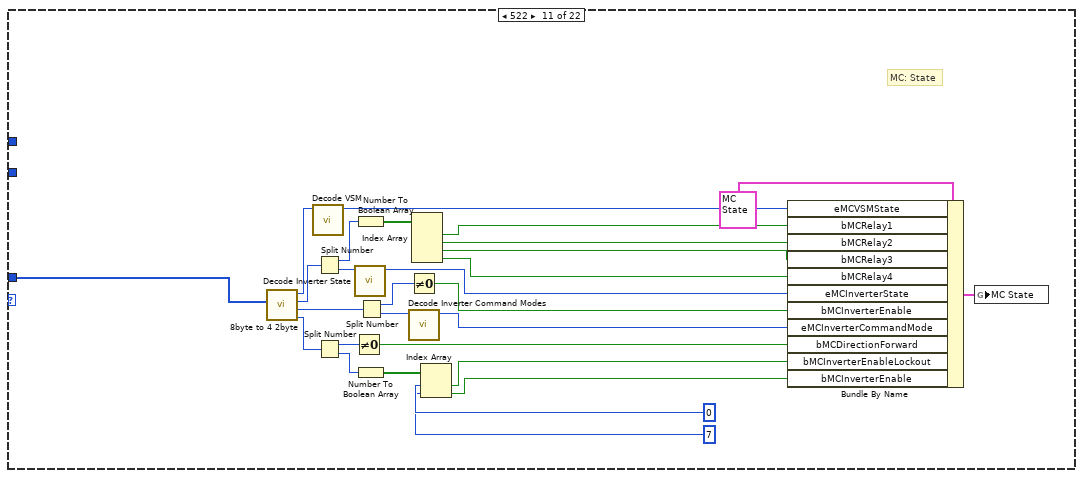
[diagram p13: hidden frame]
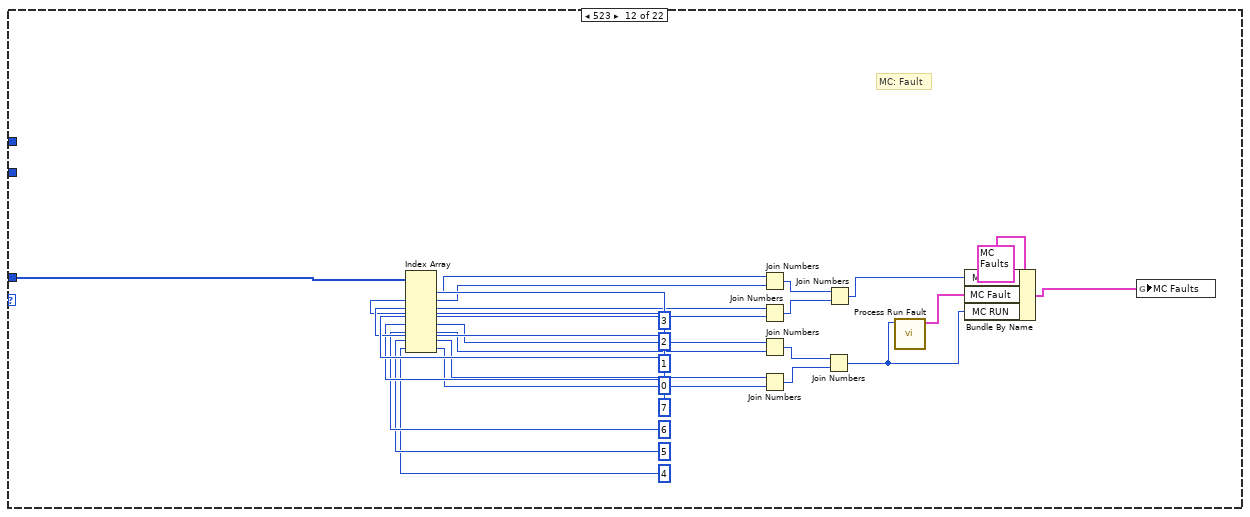
[diagram p14: hidden frame]
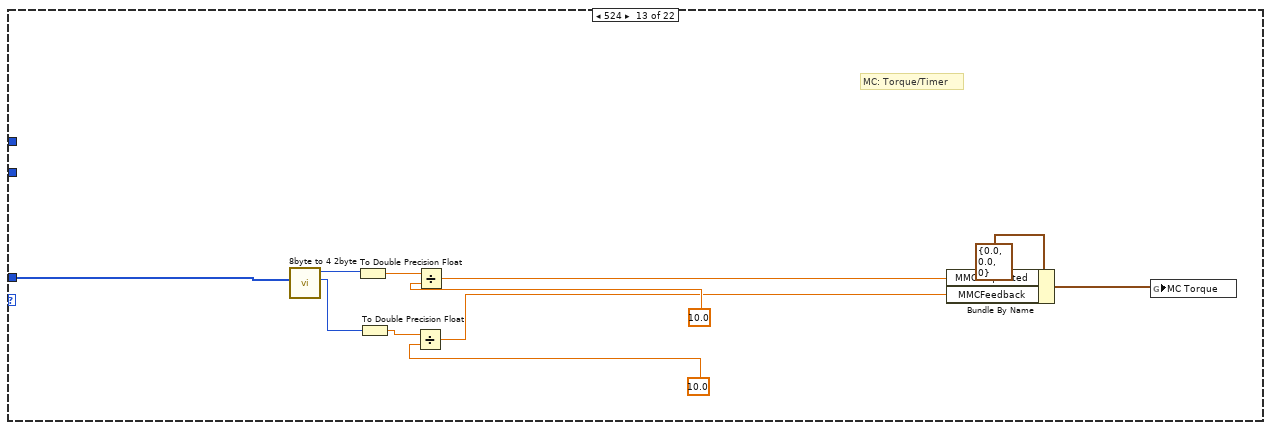
[diagram p15: hidden frame]
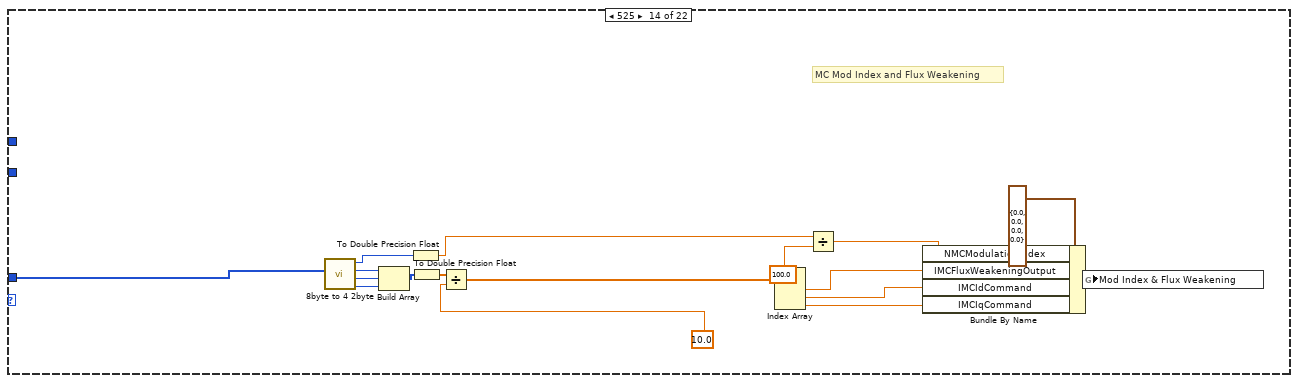
[diagram p16: hidden frame]
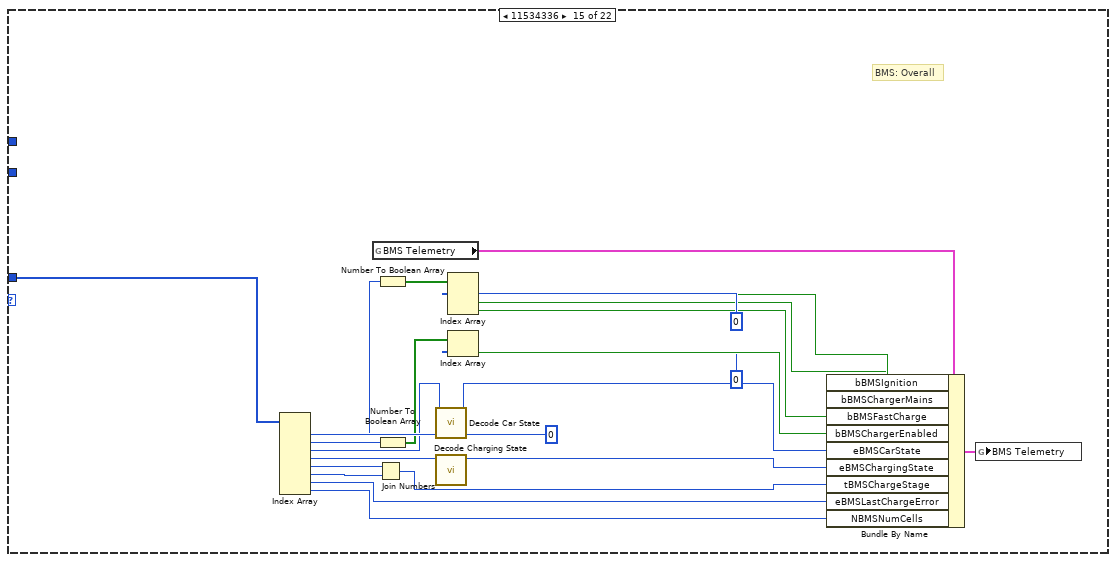
[diagram p17: hidden frame]
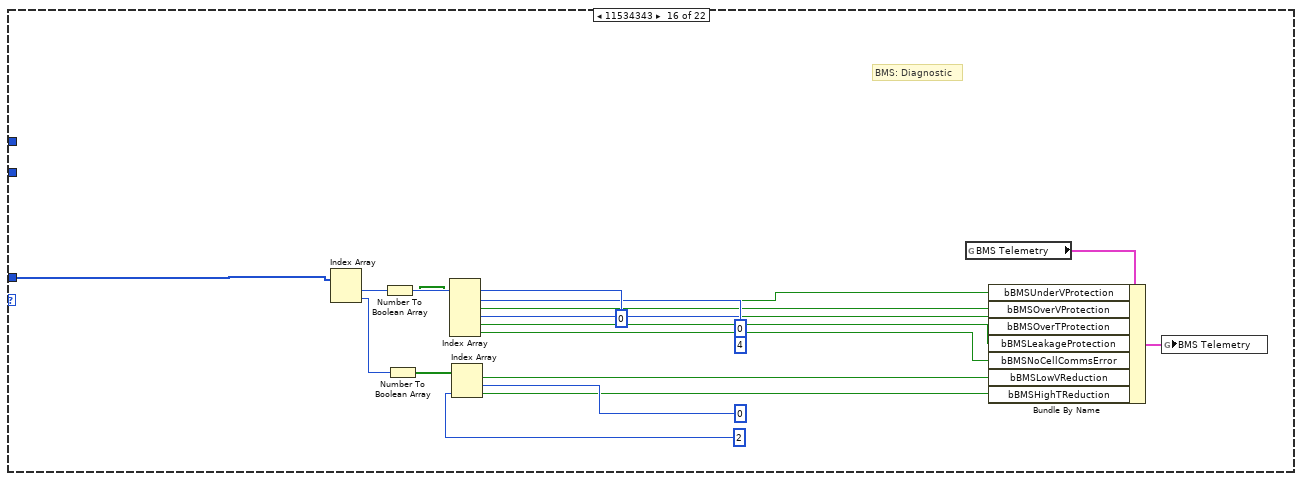
[diagram p18: hidden frame]
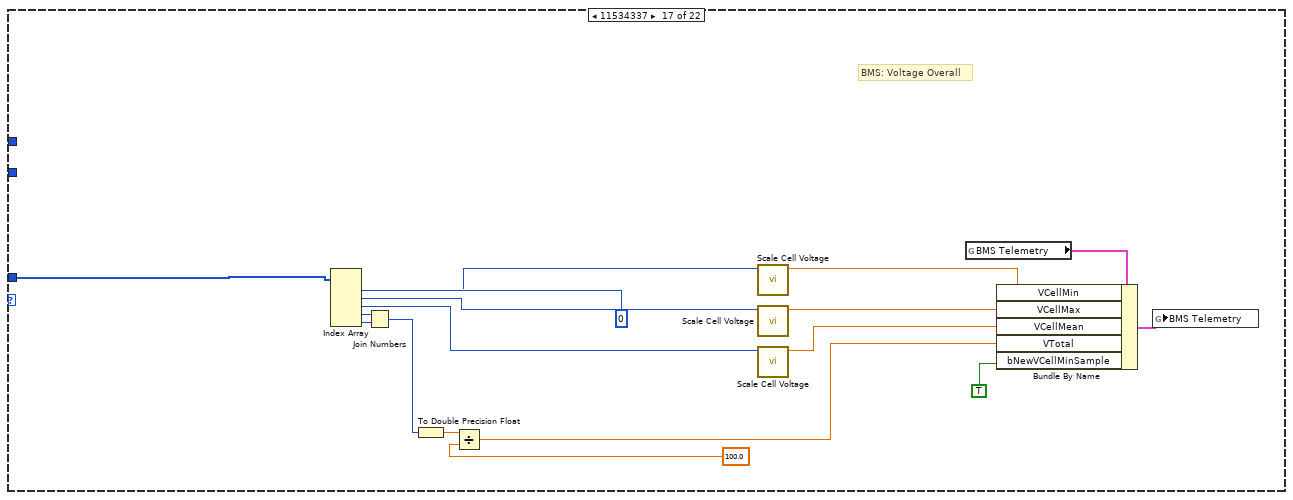
[diagram p19: hidden frame]
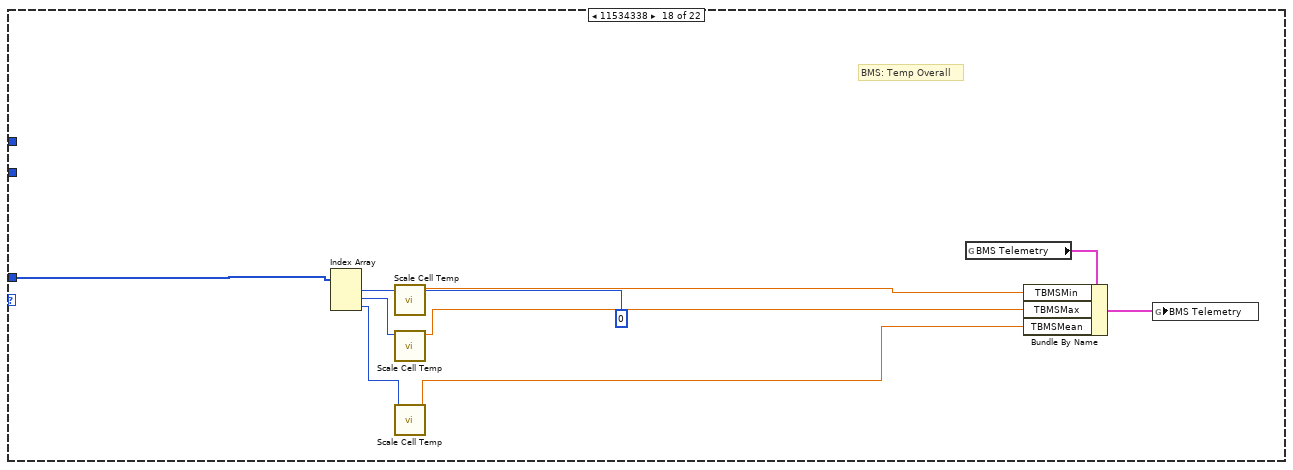
[diagram p20: hidden frame]
diagram:
  n1 = Unbundle By Name("CAN frame") -> ("identifier"=w2:u32, "payload"=w3:u8[])
  n2 = case shown="True" "Log Unique IDs" {
    tunnel: w2 -> [_ w5]
    frame False {
    }
    frame True {
      n3 = call "Find unique elements.vi"("Numeric"=w5) -> ("Array"=→"Array":u32[])  [unwired: 10 in]
    }
  }
  n4 = case shown="C00000..C00120" w2 {
    tunnel: w2 -> [_ _ _ _ _ _ _ _ _ _ _ _ _ _ _ _ _ _ w297 w325 w346 w391]
    tunnel: w3 -> [_ w8 w24 w39 w54 w73 w88 w103 w112 w124 w146 w170 w202 w212 w220 w243 w276 w286 w305 w333 w345 w383]
    tunnel: w2 -> [_ _ _ _ _ _ _ _ _ _ _ _ _ _ _ _ _ _ _ _ _ _]
    frame 0, Default {
      # "Do nothing for NULL frame"
    }
    frame 21 {
      n5 = Type Cast(type=T2 {"ButtonsBitArray"=0, "NRedRotary"=0, "NYellowRotary"=0, "NBlackRotary"=0} ("DashDriverInputs"), x=w8) -> (*(type *) &x=w7:T2)
      n6 = global write "Global Data.vi" "SDashDriverInputs"(w7) -> ()
    }
    frame 512 {
      # "MC: Temp 1"
      n7 = call "8byte to 4 2byte.vi"("payload"=w24) -> ("7,6"=w20:i16, "5,4"=w21:i16, "3,2"=w22:i16, "1,0"=w23:i16)  [unwired: 7 in]
      n8 = Build Array(w23, w22, w21, w20) -> (w13:i16[])
      n9 = To Double Precision Float(number=w13) -> (double precision float=w14:dbl[])
      n10 = Divide(x=w14, y=10.0) -> (x/y=w12:dbl[])
      n11 = Index Array(array=w12) -> (element #1=w18:dbl, element #2=w17:dbl, element #3=w16:dbl, element #4=w15:dbl)  [unwired: 4 in]
      n12 = Bundle By Name(cluster=T3 {"TMCModuleA"=0.0, "TMCModuleB"=0.0, "TMCModuleC"=0.0, "TMCGateDriver"=0.0} ("MC Temp 1"), "TMCModuleA"=w18, "TMCModuleB"=w17, "TMCModuleC"=w16, "TMCGateDriver"=w15) -> (w10:T3)
      n13 = global write "Global Data.vi" "MC Temp 1"(w10) -> ()
    }
    frame 513 {
      # "MC: Temp 2"
      n14 = call "8byte to 4 2byte.vi"("payload"=w39) -> ("7,6"=w35:i16, "5,4"=w36:i16, "3,2"=w37:i16, "1,0"=w38:i16)  [unwired: 7 in]
      n15 = Build Array(w38, w37, w36, w35) -> (w28:i16[])
      n16 = To Double Precision Float(number=w28) -> (double precision float=w29:dbl[])
      n17 = Divide(x=w29, y=10.0) -> (x/y=w27:dbl[])
      n18 = Index Array(array=w27) -> (element #1=w33:dbl, element #2=w32:dbl, element #3=w31:dbl, element #4=w30:dbl)  [unwired: 4 in]
      n19 = Bundle By Name(cluster=T4 {"TMCControlBoard"=0.0, "TMCRTD1"=0.0, "TMCRTD2"=0.0, "TMCRTD3"=0.0} ("MC Temp 2"), "TMCControlBoard"=w33, "TMCRTD1"=w32, "TMCRTD2"=w31, "TMCRTD3"=w30) -> (w26:T4)
      n20 = global write "Global Data.vi" "MC Temp 2"(w26) -> ()
    }
    frame 514 {
      # "MC: Temp 3"
      n21 = call "8byte to 4 2byte.vi"("payload"=w54) -> ("7,6"=w50:i16, "5,4"=w51:i16, "3,2"=w52:i16, "1,0"=w53:i16)  [unwired: 7 in]
      n22 = Build Array(w53, w52, w51, w50) -> (w43:i16[])
      n23 = To Double Precision Float(number=w43) -> (double precision float=w44:dbl[])
      n24 = Divide(x=w44, y=10.0) -> (x/y=w42:dbl[])
      n25 = Index Array(array=w42) -> (element #1=w48:dbl, element #2=w47:dbl, element #3=w46:dbl, element #4=w45:dbl)  [unwired: 4 in]
      n26 = Bundle By Name(cluster=T5 {"TMCRTD4"=0.0, "TMCRTD5"=0.0, "TMotor"=0.0, "MTorqueShudder"=0.0} ("MC Temp 3"), "TMCRTD4"=w48, "TMCRTD5"=w47, "TMotor"=w46, "MTorqueShudder"=w45) -> (w41:T5)
      n27 = global write "Global Data.vi" "MC Temp 3"(w41) -> ()
    }
    frame 517 {
      # "MC: Position"
      n28 = call "8byte to 4 2byte.vi"("payload"=w73) -> ("7,6"=w68:i16, "5,4"=w69:i16, "3,2"=w63:i16, "1,0"=w72:i16)  [unwired: 7 in]
      n29 = To Double Precision Float(number=w63) -> (double precision float=w62:dbl)
      n30 = Divide(x=w72, y=10.0) -> (x/y=w67:dbl)
      n31 = Divide(x=w69, y=10.0) -> (x/y=w66:dbl)
      n32 = Divide(x=w68, y=10.0) -> (x/y=w65:dbl)
      n33 = Build Array(w67, w62, w66, w65) -> (w61:dbl[])
      n34 = Index Array(array=w61) -> (element #1=w60:dbl, element #2=w59:dbl, element #3=w58:dbl, element #4=w57:dbl)  [unwired: 4 in]
      n35 = Bundle By Name(cluster=T6 {"aMotor"=0.0, "nMotor"=0.0, "fMCOutput"=0.0, "aDeltaResolverFilt"=0.0} ("MC Position"), "aMotor"=w60, "nMotor"=w59, "fMCOutput"=w58, "aDeltaResolverFilt"=w57) -> (w55:T6)
      n36 = global write "Global Data.vi" "MC Position"(w55) -> ()
    }
    frame 518 {
      # "MC: Current"
      n37 = call "8byte to 4 2byte.vi"("payload"=w88) -> ("7,6"=w84:i16, "5,4"=w85:i16, "3,2"=w86:i16, "1,0"=w87:i16)  [unwired: 7 in]
      n38 = Build Array(w87, w86, w85, w84) -> (w77:i16[])
      n39 = To Double Precision Float(number=w77) -> (double precision float=w78:dbl[])
      n40 = Divide(x=w78, y=10.0) -> (x/y=w76:dbl[])
      n41 = Index Array(array=w76) -> (element #1=w82:dbl, element #2=w81:dbl, element #3=w80:dbl, element #4=w79:dbl)  [unwired: 4 in]
      n42 = Bundle By Name(cluster=T7 {"IMCPhaseA"=0.0, "IMCPhaseB"=0.0, "IMCPhaseC"=0.0, "IMCBatteryCalc"=0.0} ("MC Current"), "IMCPhaseA"=w82, "IMCPhaseB"=w81, "IMCPhaseC"=w80, "IMCBatteryCalc"=w79) -> (w74:T7)
      n43 = global write "Global Data.vi" "MC Current"(w74) -> ()
    }
    frame 519 {
      # "MC: Voltage"
      n44 = call "8byte to 4 2byte.vi"("payload"=w103) -> ("7,6"=w99:i16, "5,4"=w100:i16, "3,2"=w101:i16, "1,0"=w102:i16)  [unwired: 7 in]
      n45 = Build Array(w102, w101, w100, w99) -> (w93:i16[])
      n46 = To Double Precision Float(number=w93) -> (double precision float=w94:dbl[])
      n47 = Divide(x=w94, y=10.0) -> (x/y=w92:dbl[])
      n48 = Index Array(array=w92) -> (element #1=w98:dbl, element #2=w97:dbl, element #3=w96:dbl, element #4=w95:dbl)  [unwired: 4 in]
      n49 = Bundle By Name(cluster=T8 {"VMCPhaseAB"=0.0, "VMCPhaseBC"=0.0, "VMCOutput"=0.0, "VMCBattery"=0.0} ("MC Voltage"), "VMCBattery"=w98, "VMCOutput"=w97, "VMCPhaseAB"=w96, "VMCPhaseBC"=w95) -> (w90:T8)
      n50 = global write "Global Data.vi" "MC Voltage"(w90) -> ()
    }
    frame 520 {
      # "MC Flux"
      n51 = call "8byte to 4 2byte.vi"("payload"=w112) -> ("7,6"=w116:i16, "5,4"=w117:i16, "3,2"=w121:i16, "1,0"=w122:i16)  [unwired: 7 in]
      n52 = Build Array(w122, w121) -> (w118:i16[])
      n53 = Build Array(w117, w116) -> (w115:i16[])
      n54 = To Double Precision Float(number=w118) -> (double precision float=w119:dbl[])
      n55 = To Double Precision Float(number=w115) -> (double precision float=w114:dbl[])
      n56 = Divide(x=w119, y=1000.0) -> (x/y=w111:dbl[])
      n57 = Divide(x=w114, y=10.0 ("7,6")) -> (x/y=w108:dbl[])
      n58 = Index Array(array=w111) -> (element #1=w110:dbl, element #2=w109:dbl)  [unwired: 2 in]
      n59 = Index Array(array=w108) -> (element #1=w107:dbl, element #2=w106:dbl)  [unwired: 2 in]
      n60 = Bundle By Name(cluster=T9 {"IMCFluxCommand"=0.0, "IMCFluxFeedback"=0.0, "IMC_Id"=0.0, "IMC_Iq"=0.0} ("MC Flux"), "IMCFluxCommand"=w110, "IMCFluxFeedback"=w109, "IMC_Id"=w107, "IMC_Iq"=w106) -> (w105:T9)
      n61 = global write "Global Data.vi" "MC Flux"(w105) -> ()
    }
    frame 521 {
      # "MC Internal Voltage"
      n62 = call "8byte to 4 2byte.vi"("payload"=w124) -> ("7,6"=w134:i16, "5,4"=w135:i16, "3,2"=w136:i16, "1,0"=w137:i16)  [unwired: 7 in]
      n63 = Build Array(w137, w136, w135, w134) -> (w128:i16[])
      n64 = To Double Precision Float(number=w128) -> (double precision float=w129:dbl[])
      n65 = Divide(x=w129, y=100.0) -> (x/y=w127:dbl[])
      n66 = Index Array(array=w127) -> (element #1=w133:dbl, element #2=w132:dbl, element #3=w131:dbl, element #4=w130:dbl)  [unwired: 4 in]
      n67 = Bundle By Name(cluster=T10 {"VMCRef1_5"=0.0, "VMCRef2_5"=0.0, "VMCRef5"=0.0, "VMCRef12"=0.0} ("MC Internal Voltages"), "VMCRef1_5"=w133, "VMCRef2_5"=w132, "VMCRef5"=w131, "VMCRef12"=w130) -> (w126:T10)
      n68 = global write "Global Data.vi" "MC Internal Voltages"(w126) -> ()
    }
    frame 522 {
      # "MC: State"
      n69 = call "8byte to 4 2byte.vi"("payload"=w146) -> ("7,6"=w154:i16, "5,4"=w161:i16, "3,2"=w164:i16, "1,0"=w165:i16)  [unwired: 7 in]
      n70 = call "Decode VSM.vi"("VSM Word"=w165) -> ("Enum"=w148:T14)  [unwired: 10 in]
      n71 = Split Number(x=w164) -> (hi(x)=w147:u8, lo(x)=w163:u8)
      n72 = Split Number(x=w154) -> (hi(x)=w141:u8, lo(x)=w158:u8)
      n73 = Not Equal To 0?(x=w141) -> (x != 0?=w140:bool)
      n74 = call "Decode Inverter State.vi"("Byte In"=w163) -> ("Inverter State Out"=w162:T12)  [unwired: 10 in]
      n75 = Number To Boolean Array(number=w147) -> (Boolean array=w153:bool[])
      n76 = Number To Boolean Array(number=w158) -> (Boolean array=w157:bool[])
      n77 = Split Number(x=w161) -> (hi(x)=w143:u8, lo(x)=w160:u8)
      n78 = Not Equal To 0?(x=w143) -> (x != 0?=w142:bool)
      n79 = call "Decode Inverter Command Modes.vi"("Numeric"=w160) -> ("Inv. Command"=w159:enum16{"CAN Mode", "VSM Mode"})  [unwired: 10 in]
      n80 = Index Array(array=w153) -> (element #1=w152:bool, element #2=w151:bool, element #3=w150:bool, element #4=w149:bool)  [unwired: 4 in]
      n81 = Index Array(array=w157, index #1=0 ("index"), index #2=7 ("index")) -> (element #1=w139:bool, element #2=w138:bool)
      n82 = Bundle By Name(cluster=T11 {"eMCInverterState"=enum."Power On", "eMCInverterRunMode"=enum."Torque Mode", "eMCInverterCommandMode"=enum."CAN Mode", "bMCInverterEnable"=FALSE, "bMCInverterEnableLockout"=FALSE, "bMCDirectionForward"=FALSE, "eMCVSMState"=enum."VSM Start", "bMCRelay1"=FALSE, "bMCRelay2"=FALSE, "bMCRelay3"=FALSE, "bMCRelay4"=FALSE} ("MC State"), "eMCVSMState"=w148, "bMCRelay1"=w152, "bMCRelay2"=w151, "bMCRelay3"=w150, "bMCRelay4"=w149, "eMCInverterState"=w162, "bMCInverterEnable"=w142, "eMCInverterCommandMode"=w159, "bMCDirectionForward"=w140, "bMCInverterEnableLockout"=w139, "bMCInverterEnable"=w138) -> (w144:T11)
      n83 = global write "Global Data.vi" "MC State"(w144) -> ()
    }
    frame 523 {
      # "MC: Fault"
      n84 = Index Array(array=w170, index #1=3 ("index"), index #2=2 ("index"), index #3=1 ("index"), index #4=0 ("index"), index #5=7 ("index"), index #6=6 ("index"), index #7=5 ("index"), index #8=4 ("index")) -> (element #1=w179:u8, element #2=w178:u8, element #3=w177:u8, element #4=w176:u8, element #5=w175:u8, element #6=w174:u8, element #7=w173:u8, element #8=w172:u8)
      n85 = Join Numbers(hi=w179, lo=w178) -> ((hi.lo)=w180:u16)
      n86 = Join Numbers(hi=w177, lo=w176) -> ((hi.lo)=w181:u16)
      n87 = Join Numbers(hi=w175, lo=w174) -> ((hi.lo)=w182:u16)
      n88 = Join Numbers(hi=w173, lo=w172) -> ((hi.lo)=w183:u16)
      n89 = Join Numbers(hi=w182, lo=w183) -> ((hi.lo)=w166:u32)
      n90 = Join Numbers(hi=w180, lo=w181) -> ((hi.lo)=w171:u32)
      n91 = call "Process Run Fault.vi"("RUN Fault"=w166) -> ("MC Fault"=w167:T18)  [unwired: 10 in]
      n92 = Bundle By Name(cluster=T15 {"MC Fault"={"Over-Speed"=FALSE, "Over-Current"=FALSE, "Over-Voltage"=FALSE, "Inverter Over-Temp"=FALSE, "Direction Command"=FALSE, "Inverter Response Time-Out"=FALSE, "Desat Fault"=FALSE, "Hardware Over-Current"=FALSE, "Under-Voltage"=FALSE, "CAN Command Message Lost"=FALSE, "Motor Over-Temp"=FALSE, "Module A Over-Temp"=FALSE, "Module B Over-Temp"=FALSE, "Module C Over-Temp"=FALSE, "PCB Over-Temp"=FALSE, "Gate Driver 1 Over-Temp"=FALSE, "Gate Driver 2 Over-Temp"=FALSE, "Gate Drive 3 Over-Temp"=FALSE, "Current Sensor Fault"=FALSE, "Resolver Not Connected"=FALSE}, "MC Post"=0, "MC RUN"=0} ("MC Faults"), "MC Post"=w171, "MC Fault"=w167, "MC RUN"=w166) -> (w168:T15)
      n93 = global write "Global Data.vi" "MC Faults"(w168) -> ()
    }
    frame 524 {
      # "MC: Torque/Timer"
      n94 = call "8byte to 4 2byte.vi"("payload"=w202) -> ("3,2"=w198:i16, "1,0"=w201:i16)  [unwired: 7 in, 2 out]
      n95 = To Double Precision Float(number=w201) -> (double precision float=w200:dbl)
      n96 = To Double Precision Float(number=w198) -> (double precision float=w197:dbl)
      n97 = Divide(x=w197, y=10.0) -> (x/y=w194:dbl)
      n98 = Divide(x=w200, y=10.0) -> (x/y=w195:dbl)
      n99 = Bundle By Name(cluster=T16 {"MMCRequested"=0.0, "MMCFeedback"=0.0, "tMCElapsed"=0} ("MC Torque"), "MMCRequested"=w195, "MMCFeedback"=w194) -> (w193:T16)
      n100 = global write "Global Data.vi" "MC Torque"(w193) -> ()
    }
    frame 525 {
      # "MC Mod Index and Flux Weakening"
      n101 = call "8byte to 4 2byte.vi"("payload"=w212) -> ("7,6"=w215:i16, "5,4"=w214:i16, "3,2"=w213:i16, "1,0"=w206:i16)  [unwired: 7 in]
      n102 = Build Array(w213, w214, w215) -> (w217:i16[])
      n103 = To Double Precision Float(number=w206) -> (double precision float=w205:dbl)
      n104 = To Double Precision Float(number=w217) -> (double precision float=w216:dbl[])
      n105 = Divide(x=w216, y=10.0) -> (x/y=w218:dbl[])
      n106 = Index Array(array=w218) -> (element #1=w209:dbl, element #2=w208:dbl, element #3=w207:dbl)  [unwired: 3 in]
      n107 = Divide(x=w205, y=100.0) -> (x/y=w203:dbl)
      n108 = Bundle By Name(cluster=T17 {"NMCModulationIndex"=0.0, "IMCFluxWeakeningOutput"=0.0, "IMCIdCommand"=0.0, "IMCIqCommand"=0.0} ("Mod Index & Flux Weakening"), "NMCModulationIndex"=w203, "IMCFluxWeakeningOutput"=w209, "IMCIdCommand"=w208, "IMCIqCommand"=w207) -> (w211:T17)
      n109 = global write "Global Data.vi" "Mod Index & Flux Weakening"(w211) -> ()
    }
    frame 11534336 {
      # "BMS: Overall"
      n110 = Index Array(array=w220, index #1=0 ("index")) -> (element #1=w239:u8, element #2=w233:u8, element #3=w228:u8, element #4=w227:u8, element #5=w225:u8, element #6=w224:u8, element #7=w222:u8, element #8=w221:u8)  [unwired: 7 in]
      n111 = global read "Global Data.vi" "BMS Telemetry"() -> (w242:T19)
      n112 = Join Numbers(hi=w225, lo=w224) -> ((hi.lo)=w223:u16)
      n113 = Number To Boolean Array(number=w239) -> (Boolean array=w238:bool[])
      n114 = Number To Boolean Array(number=w233) -> (Boolean array=w231:bool[])
      n115 = call "Decode Car State.vi"("Numeric"=w228) -> ("Car State"=w229:T20)  [unwired: 10 in]
      n116 = call "Decode Charging State.vi"("Numeric"=w227) -> ("Charging State"=w226:T21)  [unwired: 10 in]
      n117 = Index Array(array=w238, index #1=0 ("index")) -> (element #1=w236:bool, element #2=w235:bool, element #3=w234:bool)  [unwired: 2 in]
      n118 = Index Array(array=w231, index=0) -> (element=w232:bool)
      n119 = Bundle By Name(cluster=w242, "bBMSIgnition"=w236, "bBMSChargerMains"=w235, "bBMSFastCharge"=w234, "bBMSChargerEnabled"=w232, "eBMSCarState"=w229, "eBMSChargingState"=w226, "tBMSChargeStage"=w223, "eBMSLastChargeError"=w222, "NBMSNumCells"=w221) -> (w241:T19)
      n120 = global write "Global Data.vi" "BMS Telemetry"(w241) -> ()
    }
    frame 11534343 {
      # "BMS: Diagnostic"
      n121 = Index Array(array=w243, index #1=0 ("index")) -> (element #1=w258:u8, element #2=w249:u8)  [unwired: 1 in]
      n122 = Number To Boolean Array(number=w258) -> (Boolean array=w257:bool[])
      n123 = Number To Boolean Array(number=w249) -> (Boolean array=w248:bool[])
      n124 = Index Array(array=w257, index #1=0 ("index"), index #3=4 ("index")) -> (element #1=w255:bool, element #2=w254:bool, element #3=w252:bool, element #4=w251:bool, element #5=w250:bool)  [unwired: 3 in]
      n125 = Index Array(array=w248, index #1=0 ("index"), index #2=2 ("index")) -> (element #1=w245:bool, element #2=w244:bool)
      n126 = global read "Global Data.vi" "BMS Telemetry"() -> (w261:T19)
      n127 = Bundle By Name(cluster=w261, "bBMSUnderVProtection"=w255, "bBMSOverVProtection"=w254, "bBMSOverTProtection"=w252, "bBMSLeakageProtection"=w251, "bBMSNoCellCommsError"=w250, "bBMSLowVReduction"=w245, "bBMSHighTReduction"=w244) -> (w260:T19)
      n128 = global write "Global Data.vi" "BMS Telemetry"(w260) -> ()
    }
    frame 11534337 {
      # "BMS: Voltage Overall"
      n129 = Index Array(array=w276, index #1=0 ("index")) -> (element #1=w274:u8, element #2=w273:u8, element #3=w272:u8, element #4=w271:u8, element #5=w270:u8)  [unwired: 4 in]
      n130 = Join Numbers(hi=w271, lo=w270) -> ((hi.lo)=w269:u16)
      n131 = To Double Precision Float(number=w269) -> (double precision float=w268:dbl)
      n132 = Divide(x=w268, y=100.0) -> (x/y=w263:dbl)
      n133 = call "Scale Cell Voltage.vi"("Numeric in"=w274) -> ("Numeric out"=w266:dbl)  [unwired: 10 in]
      n134 = call "Scale Cell Voltage.vi"("Numeric in"=w273) -> ("Numeric out"=w265:dbl)  [unwired: 10 in]
      n135 = call "Scale Cell Voltage.vi"("Numeric in"=w272) -> ("Numeric out"=w264:dbl)  [unwired: 10 in]
      n136 = global read "Global Data.vi" "BMS Telemetry"() -> (w278:T19)
      n137 = Bundle By Name(cluster=w278, "VCellMin"=w266, "VCellMax"=w265, "VCellMean"=w264, "VTotal"=w263, "bNewVCellMinSample"=TRUE) -> (w277:T19)
      n138 = global write "Global Data.vi" "BMS Telemetry"(w277) -> ()
    }
    frame 11534338 {
      # "BMS: Temp Overall"
      n139 = Index Array(array=w286, index #1=0 ("index")) -> (element #1=w284:u8, element #2=w283:u8, element #3=w282:u8)  [unwired: 2 in]
      n140 = call "Scale Cell Temp.vi"("Numeric in"=w284) -> ("Numeric out"=w281:dbl)  [unwired: 10 in]
      n141 = call "Scale Cell Temp.vi"("Numeric in"=w283) -> ("Numeric out"=w280:dbl)  [unwired: 10 in]
      n142 = call "Scale Cell Temp.vi"("Numeric in"=w282) -> ("Numeric out"=w279:dbl)  [unwired: 10 in]
      n143 = global read "Global Data.vi" "BMS Telemetry"() -> (w288:T19)
      n144 = Bundle By Name(cluster=w288, "TBMSMin"=w281, "TBMSMax"=w280, "TBMSMean"=w279) -> (w287:T19)
      n145 = global write "Global Data.vi" "BMS Telemetry"(w287) -> ()
    }
    frame 11534592..11534847 {
      # "BMS: Cell Voltages"
      n146 = Split Number(x=w297) -> (lo(x)=w296:u16)  [unwired: 1 out]
      n147 = Index Array(array=w305, index #1=0 ("index")) -> (element #1=w292:u8, element #2=w304:u8, element #3=w303:u8, element #4=w302:u8, element #5=w301:u8, element #6=w300:u8, element #7=w299:u8)  [unwired: 7 in, 1 out]
      n148 = Split Number(x=w296) -> (lo(x)=w294:u8)  [unwired: 1 out]
      n149 = To Long Integer(number=w294) -> (32bit integer=w293:i32)
      n150 = Build Array(w292, w292, w304, w303, w302, w301, w300, w299) -> (w290:u8[])
      n151 = Multiply(x=w293, y=8) -> (x*y=w289:i32)
      n152 = Array Max & Min(array=w290) -> (max value=w291:u8)  [unwired: 3 out]
      n153 = case shown="2..255, Default" w291 {
        tunnel: w290 -> [_ w308]
        tunnel: w289 -> [_ w306]
        frame 0, 1 {
        }
        frame 2..255, Default {
          n154 = global read "Global Data.vi" "BMS Telemetry"() -> (w309:T19)
          n155 = for {
            tunnel: w308 -> [w315] mode=indexing
            tunnel: [w316] -> w307 mode=indexing
            n156 = call "Scale Cell Voltage.vi"("Numeric in"=w315) -> ("Numeric out"=w316:dbl)  [unwired: 10 in]
          }
          n157 = Unbundle By Name(w309) -> ("VCells"=w312:T22)
          n158 = Cluster To Array(cluster=w312) -> (array=w311:dbl[])
          n159 = Replace Array Subset(array=w311, new element=w307, index=w306) -> (w313:dbl[])
          n160 = Array To Cluster(array=w313) -> (cluster=w314:T23)
          n161 = Bundle By Name(cluster=w309, "VCells"=w314) -> (w310:T19)
          n162 = global write "Global Data.vi" "BMS Telemetry"(w310) -> ()
        }
      }
    }
    frame 11534848..11535103 {
      # "BMS: Cell Temperatures"
      n163 = Split Number(x=w325) -> (lo(x)=w324:u16)  [unwired: 1 out]
      n164 = Index Array(array=w333, index #1=0 ("index")) -> (element #1=w320:u8, element #2=w332:u8, element #3=w331:u8, element #4=w330:u8, element #5=w329:u8, element #6=w328:u8, element #7=w327:u8)  [unwired: 7 in, 1 out]
      n165 = Split Number(x=w324) -> (lo(x)=w322:u8)  [unwired: 1 out]
      n166 = To Long Integer(number=w322) -> (32bit integer=w321:i32)
      n167 = Build Array(w320, w320, w332, w331, w330, w329, w328, w327) -> (w318:u8[])
      n168 = Multiply(x=w321, y=8) -> (x*y=w317:i32)
      n169 = Array Max & Min(array=w318) -> (max value=w319:u8)  [unwired: 3 out]
      n170 = case shown="2..255, Default" w319 {
        tunnel: w318 -> [_ w336]
        tunnel: w317 -> [_ w334]
        frame 0, 1 {
        }
        frame 2..255, Default {
          n171 = global read "Global Data.vi" "BMS Telemetry"() -> (w337:T19)
          n172 = for {
            tunnel: w336 -> [w343] mode=indexing
            tunnel: [w344] -> w335 mode=indexing
            n173 = call "Scale Cell Temp.vi"("Numeric in"=w343) -> ("Numeric out"=w344:dbl)  [unwired: 10 in]
          }
          n174 = Unbundle By Name(w337) -> ("TBMSCells"=w340:T24)
          n175 = Cluster To Array(cluster=w340) -> (array=w339:dbl[])
          n176 = Replace Array Subset(array=w339, new element=w335, index=w334) -> (w341:dbl[])
          n177 = Array To Cluster(array=w341) -> (cluster=w342:T25)
          n178 = Bundle By Name(cluster=w337, "TBMSCells"=w342) -> (w338:T19)
          n179 = global write "Global Data.vi" "BMS Telemetry"(w338) -> ()
        }
      }
    }
    frame 11535104..11535359 {
      # "indexes information at 0"
      # "mult by 8 to index\narray correctly"
      # "Remove all but last byte"
      # "BMS Balancing"
      n180 = Split Number(x=w346) -> (lo(x)=w354:u16)  [unwired: 1 out]
      n181 = Index Array(array=w345, index #1=0 ("index")) -> (element #1=w350:u8, element #2=w361:u8, element #3=w360:u8, element #4=w359:u8, element #5=w358:u8, element #6=w357:u8, element #7=w356:u8)  [unwired: 7 in, 1 out]
      n182 = Split Number(x=w354) -> (lo(x)=w352:u8)  [unwired: 1 out]
      n183 = To Long Integer(number=w352) -> (32bit integer=w351:i32)
      n184 = Build Array(w350, w350, w361, w360, w359, w358, w357, w356) -> (w348:u8[])
      n185 = Multiply(x=w351, y=8) -> (x*y=w347:i32)
      n186 = Array Max & Min(array=w348) -> (max value=w349:u8)  [unwired: 3 out]
      n187 = case shown="2..255, Default" w349 {
        tunnel: w348 -> [_ w364]
        tunnel: w347 -> [_ w362]
        frame 0, 1 {
        }
        frame 2..255, Default {
          # "push back into cluster"
          # "replace values in cluster\nat indexed position"
          n188 = global read "Global Data.vi" "BMS Telemetry"() -> (w365:T19)
          n189 = for {
            tunnel: w364 -> [w372] mode=indexing
            tunnel: [w371] -> w363 mode=indexing
            # "scale each value"
            n190 = call "Scale Cell Balance.vi"("Numeric in"=w372) -> ("Numeric Out"=w371:dbl)  [unwired: 10 in]
          }
          n191 = Unbundle By Name(w365) -> ("BCells"=w368:T26)
          n192 = Cluster To Array(cluster=w368) -> (array=w367:dbl[])
          n193 = Replace Array Subset(array=w367, new element=w363, index=w362) -> (w369:dbl[])
          n194 = Array To Cluster(array=w369) -> (cluster=w370:T27)
          n195 = Bundle By Name(cluster=w365, "BCells"=w370) -> (w366:T19)
          n196 = global write "Global Data.vi" "BMS Telemetry"(w366) -> ()
        }
      }
    }
    frame 12582912..12583200 {
      # "gets the battery group index"
      # "Processes  the CAN Temp \nboard Data"
      # "Conmbines 1 byte elements\ninto 2 byte elements\nTakes in low then hi, order is \nswitched on exit"
      n197 = Split Number(x=w391) -> (lo(x)=w390:u16)  [unwired: 1 out]
      n198 = Index Array(array=w383, index #1=0 ("index")) -> (element #1=w382:u8, element #2=w381:u8, element #3=w380:u8, element #4=w379:u8, element #5=w378:u8, element #6=w377:u8, element #7=w376:u8, element #8=w375:u8)  [unwired: 7 in]
      n199 = To Long Integer(number=w390) -> (32bit integer=w392:i32)
      n200 = Join Numbers(hi=w381, lo=w382) -> ((hi.lo)=w387:u16)
      n201 = Join Numbers(hi=w379, lo=w380) -> ((hi.lo)=w386:u16)
      n202 = Join Numbers(hi=w377, lo=w378) -> ((hi.lo)=w385:u16)
      n203 = Join Numbers(hi=w375, lo=w376) -> ((hi.lo)=w384:u16)
      n204 = Build Array(w387, w386, w385, w384) -> (w388:u16[])
      n205 = Multiply(x=w392, y=4) -> (x*y=w374:i32)
      n206 = Array Max & Min(array=w388) -> ()  [unwired: 4 out]
      n207 = case shown="True" TRUE {
        tunnel: w388 -> [_ w407]
        tunnel: w374 -> [_ w395]
        tunnel: [_ w395] -> _
        frame False {
        }
        frame True {
          w398 = T28 {0.0, 0.0, 0.0, 0.0, 0.0, 0.0, 0.0, 0.0, 0.0, 0.0, 0.0, 0.0, 0.0, 0.0, 0.0, 0.0, 0.0, 0.0, 0.0, 0.0, 0.0, 0.0, 0.0, 0.0, 0.0, 0.0, 0.0, 0.0, 0.0, 0.0, 0.0, 0.0, 0.0, 0.0, 0.0, 0.0, 0.0, 0.0, 0.0, 0.0, 0.0, 0.0, 0.0, 0.0, 0.0, 0.0, 0.0, 0.0, 0.0, 0.0, 0.0, 0.0, 0.0, 0.0, 0.0, 0.0, 0.0, 0.0, 0.0, 0.0, 0.0, 0.0, 0.0, 0.0, 0.0, 0.0, 0.0, 0.0, 0.0, 0.0, 0.0, 0.0, 0.0, 0.0, 0.0, 0.0, 0.0, 0.0, 0.0, 0.0, 0.0, 0.0, 0.0, 0.0, 0.0, 0.0, 0.0, 0.0, 0.0, 0.0, 0.0, 0.0, 0.0, 0.0, 0.0, 0.0, 0.0, 0.0, 0.0, 0.0, 0.0, 0.0, 0.0, 0.0, 0.0, 0.0, 0.0, 0.0, 0.0, 0.0, 0.0, 0.0, 0.0, 0.0, 0.0, 0.0, 0.0, 0.0, 0.0, 0.0, 0.0, 0.0, 0.0, 0.0, 0.0, 0.0, 0.0, 0.0, 0.0, 0.0, 0.0, 0.0, 0.0, 0.0, 0.0, 0.0, 0.0, 0.0, 0.0, 0.0, 0.0, 0.0, 0.0, 0.0, 0.0, 0.0, 0.0, 0.0, 0.0, 0.0, 0.0, 0.0, 0.0, 0.0, 0.0, 0.0, 0.0, 0.0, 0.0, 0.0, 0.0, 0.0, 0.0, 0.0, 0.0, 0.0, 0.0, 0.0, 0.0, 0.0, 0.0, 0.0, 0.0, 0.0, 0.0, 0.0, 0.0, 0.0, 0.0, 0.0, 0.0, 0.0, 0.0, 0.0, 0.0, 0.0, 0.0, 0.0, 0.0, 0.0, 0.0, 0.0, 0.0, 0.0, 0.0, 0.0, 0.0, 0.0, 0.0, 0.0, 0.0, 0.0, 0.0, 0.0, 0.0, 0.0, 0.0, 0.0, 0.0, 0.0, 0.0, 0.0, 0.0, 0.0, 0.0, 0.0, 0.0, 0.0, 0.0, 0.0, 0.0, 0.0, 0.0, 0.0, 0.0, 0.0, 0.0, 0.0, 0.0, 0.0, 0.0, 0.0, 0.0, 0.0, 0.0, 0.0, 0.0, 0.0, 0.0, 0.0, 0.0, 0.0, 0.0, 0.0, 0.0, 0.0, 0.0, 0.0, 0.0, 0.0, 0.0, 0.0, 0.0, 0.0, 0.0, 0.0, 0.0, 0.0, 0.0, 0.0, 0.0, 0.0, 0.0, 0.0, 0.0, 0.0, 0.0, 0.0, 0.0, 0.0, 0.0, 0.0, 0.0, 0.0, 0.0, 0.0, 0.0, 0.0, 0.0, 0.0, 0.0, 0.0, 0.0, 0.0, 0.0, 0.0, 0.0, 0.0}
          # "calculates average"
          # "allows an array over 256\nto be created"
          # "Converts CAN Message\nto temp"
          n208 = for {
            N: 4 -> [_]
            tunnel: w407 -> [w414] mode=indexing
            tunnel: [w415] -> w403 mode=indexing
            n209 = Subtract(x=w414, y=60) -> (x-y=w412:i32)
            n210 = call "Scale Can Temp.vi"("Numeric"=w412) -> ("Double out"=w416:dbl)  [unwired: 10 in]
            n211 = call "Calculate Thermistor Temp.vi"("Numeric"=w416) -> ("Numeric 2"=w415:dbl)  [unwired: 10 in]
          }
          n212 = global read "Global Data.vi" "BMS Telemetry"() -> (w410:T19)
          n213 = Unbundle By Name(w410) -> ("Battery Temp"=w411:T29)
          n214 = Cluster To Array(cluster=w411) -> (array=w408:dbl[])
          n215 = Replace Array Subset(array=w408, new element=w403, index=w395) -> (w401:dbl[])
          n216 = Add Array Elements(numeric array=w401) -> (sum=w402:dbl)
          n217 = Divide(x=w402, y=288.0) -> (x/y=w404:dbl)
          n218 = Array Max & Min(array=w401) -> (max value=w400:dbl, min value=w399:dbl)  [unwired: 2 out]
          n219 = Type Cast(type=w398, x=w401) -> (*(type *) &x=w397:T28)
          n220 = Select(t=w398, s="Reset Array", f=w397) -> (s? t:f=w396:T28)
          n221 = Bundle By Name(cluster=w410, "Battery Temp"=w396, "TCellMax"=w400, "TCellMin"=w399, "TCellMean"=w404) -> (w406:T19)
          n222 = global write "Global Data.vi" "BMS Telemetry"(w406) -> ()
        }
      }
    }
  }
